vi "Telemetry2022_2.vi"() -> ()   [LabVIEW 2017]
uses:
  <vilib>/xnet/xnet.llb/XNET Frame CAN.ctl
  <vilib>/xnet/xnet.llb/XNET Frame Type CAN.ctl
  <vilib>/xnet/xnet.llb/XNET Read (Frame CAN).vi
panel:
  out "819":dbl[](array[numeric])
  out "513":dbl[](array[numeric])
  out "390":dbl[](array[numeric])
  out "389":dbl[](array[numeric])
  out "376":dbl[](array[numeric])
  out "647":dbl[](array[numeric])
  out "644":dbl[](array[numeric])
  out "645":dbl[](array[numeric])
  out "646":dbl[](array[numeric])
  out "401":dbl
  out "394":T1
  out "393":T2
  out "532":T3
  out "530":T4
  out "651":T5
  out "650":T6
  out "649":T7
  out "648":T8
  in  "ip":string="127.0.0.1"
  out "UDP timestep":u32(graph)
  out "Frames to update this timestep":u32[](array[numeric])
  in  "stresstest":bool
  out "Actual Timestep":u32(graph)
  out "105":T9
  out "1029":T10
  out "1157":T11
  out "1153":T12
  out "1030":T13
  out "873":T14
  out "820":T15
  in  "stresstest2":u8[][](array[numeric])=[[2, 132, 0, 0, 0, 0, 0, 0, 0, 0], [2, 133, 0, 0, 0, 0, 0, 0, 0, 0], [2, 134, 0, 0, 0, 0, 0, 0, 0, 0], [2, 135, 0, 0, 0, 0, 0, 0, 0, 0], [1, 116, 0, 0, 0, 0, 0, 0, 0, 0], [1, 120, 0, 0, 0, 0, 0, 0, 0, 0], [1, 133, 0, 0, 0, 0, 0, 0, 0, 0], [1, 134, 0, 0, 0, 0, 0, 0, 0, 0], [2, 1, 0, 0, 0, 0, 0, 0, 0, 0], [2, 0, 0, 0, 0, 0, 0, 0, 0, 0], [5, 129, 0, 0, 0, 0, 0, 0, 0, 0], [3, 51, 0, 0, 0, 0, 0, 0, 0, 0], [3, 52, 0, 0, 0, 0, 0, 0, 0, 0], [3, 105, 0, 0, 0, 0, 0, 0, 0, 0], [4, 6, 0, 0, 0, 0, 0, 0, 0, 0], [4, 129, 0, 0, 0, 0, 0, 0, 0, 0], [4, 133, 0, 0, 0, 0, 0, 0, 0, 0], [4, 5, 0, 0, 0, 0, 0, 0, 0, 0], [0, 105, 0, 0, 0, 0, 0, 0, 0, 0], [2, 136, 0, 0, 0, 0, 0, 0, 0, 0], [2, 137, 0, 0, 0, 0, 0, 0, 0, 0], [2, 138, 0, 0, 0, 0, 0, 0, 0, 0], [2, 139, 0, 0, 0, 0, 0, 0, 0, 0], [2, 18, 0, 0, 0, 0, 0, 0, 0, 0], [2, 20, 0, 0, 0, 0, 0, 0, 0, 0], [1, 137, 0, 0, 0, 0, 0, 0, 0, 0], [1, 138, 0, 0, 0, 0, 0, 0, 0, 0], [1, 145, 0, 0, 0, 0, 0, 0, 0, 0]]
  in  "stresstest1":u8[][](array[numeric])=[[2, 132, 1, 0, 1, 0, 1, 0, 1, 0], [2, 133, 1, 0, 1, 0, 1, 0, 1, 0], [2, 134, 1, 0, 1, 0, 1, 0, 1, 0], [2, 135, 1, 0, 1, 0, 1, 0, 1, 0], [1, 116, 0, 0, 0, 0, 1, 0, 0, 0], [1, 120, 1, 0, 0, 0, 1, 0, 0, 0], [1, 133, 0, 15, 1, 0, 1, 0, 1, 0], [1, 134, 0, 15, 1, 0, 1, 0, 1, 0], [2, 1, 1, 0, 1, 0, 1, 0, 1, 0], [2, 0, 1, 0, 1, 0, 1, 0, 1, 0], [5, 129, 1, 0, 0, 0, 0, 0, 0, 0], [3, 51, 255, 255, 255, 255, 255, 255, 255, 255], [3, 52, 255, 255, 255, 255, 255, 255, 255, 255], [3, 105, 1, 1, 1, 1, 1, 0, 0, 0], [4, 6, 0, 1, 0, 1, 0, 1, 0, 1], [4, 129, 255, 255, 255, 255, 255, 255, 255, 255], [4, 133, 255, 255, 255, 255, 255, 255, 255, 255], [4, 5, 0, 1, 0, 1, 0, 1, 0, 1], [0, 105, 0, 0, 0, 1, 1, 1, 128, 1], [2, 136, 1, 0, 1, 0, 1, 0, 1, 0], [2, 137, 1, 0, 1, 0, 1, 0, 1, 0], [2, 138, 1, 0, 1, 0, 1, 0, 1, 0], [2, 139, 1, 0, 1, 0, 1, 0, 1, 0], [2, 18, 255, 255, 255, 255, 255, 255, 255, 255], [2, 20, 1, 0, 1, 0, 1, 0, 1, 0], [1, 137, 1, 0, 1, 0, 1, 0, 1, 0], [1, 138, 1, 0, 1, 0, 1, 0, 1, 0], [1, 145, 2, 0, 0, 0, 0, 0, 0, 0]]
  out "1409":dbl
  out "512":T16
  out "372":dbl
  out "?":T17(tab)
  in  "?":bool
  out "CAN2 Frame to signal":errorcluster
  out "XNET error (CAN3)":errorcluster
  out "XNET error (CAN2)":errorcluster
  out "NI-CAN1 error":errorcluster {"code" format="%.0x"}
  out "NI-CAN0 error":errorcluster {"code" format="%.0x"}
  out "CAN1 Frame to signal":errorcluster
  out "UDP Read error":errorcluster
  in  "Data source":u16(ring) items=["WiFi-UDP", "XNET-USB", "CAN-USB", "Log Replay"]
  in  "Port":u16=23456
  in  "Main timestep":u32=10
  out "Key Navigation error":errorcluster
  out "Is running":bool
  out "Key":T18(ring)
  in  "Reset Keyboard":bool
  out "all signal data":dbl[](array[numeric])
  out "rec array":u8[][](array[numeric])=[[2, 225, 14, 196, 12, 0, 0, 0, 0, 0], [2, 226, 35, 253, 12, 0, 0, 0, 0, 0], [2, 227, 56, 248, 12, 0, 0, 0, 0, 0], [2, 228, 77, 195, 12, 0, 0, 0, 0, 0], [2, 241, 7, 28, 0, 0, 0, 0, 0, 0], [2, 242, 14, 27, 0, 0, 0, 0, 0, 0], [2, 243, 21, 29, 0, 0, 0, 0, 0, 0], [2, 244, 28, 28, 0, 0, 0, 0, 0, 0], [0, 144, 12, 42, 12, 247, 12, 20, 12, 129], [0, 112, 11, 37, 0, 225, 1, 0, 0, 0], [0, 113, 15, 104, 8, 4, 1, 0, 0, 0], [2, 0, 2, 4, 5, 5, 2, 0, 0, 0], [0, 98, 3, 242, 1, 24, 0, 131, 0, 0], [0, 99, 46, 33, 1, 1, 1, 1, 1, 44], [0, 102, 2, 71, 1, 51, 0, 74, 0, 0], [0, 103, 33, 35, 1, 1, 1, 1, 1, 44]]
  out "frame data":T19[](array[typedef]) {"payload" format="%x"; "timestamp" format="%<%.7X\n%x>T"; "type" items=["CAN Data"=0, "CAN Remote"=1, "CAN Bus Error"=2, "CAN 2.0 Data"=8, "CAN FD Data"=16, "CAN FD+BRS Data"=24, "J1939 Data"=192, "Delay"=224, "Log Trigger"=225, "Start Trigger"=226]; "identifier" format="%x"}
  # "CAN1"
  # "CAN2"
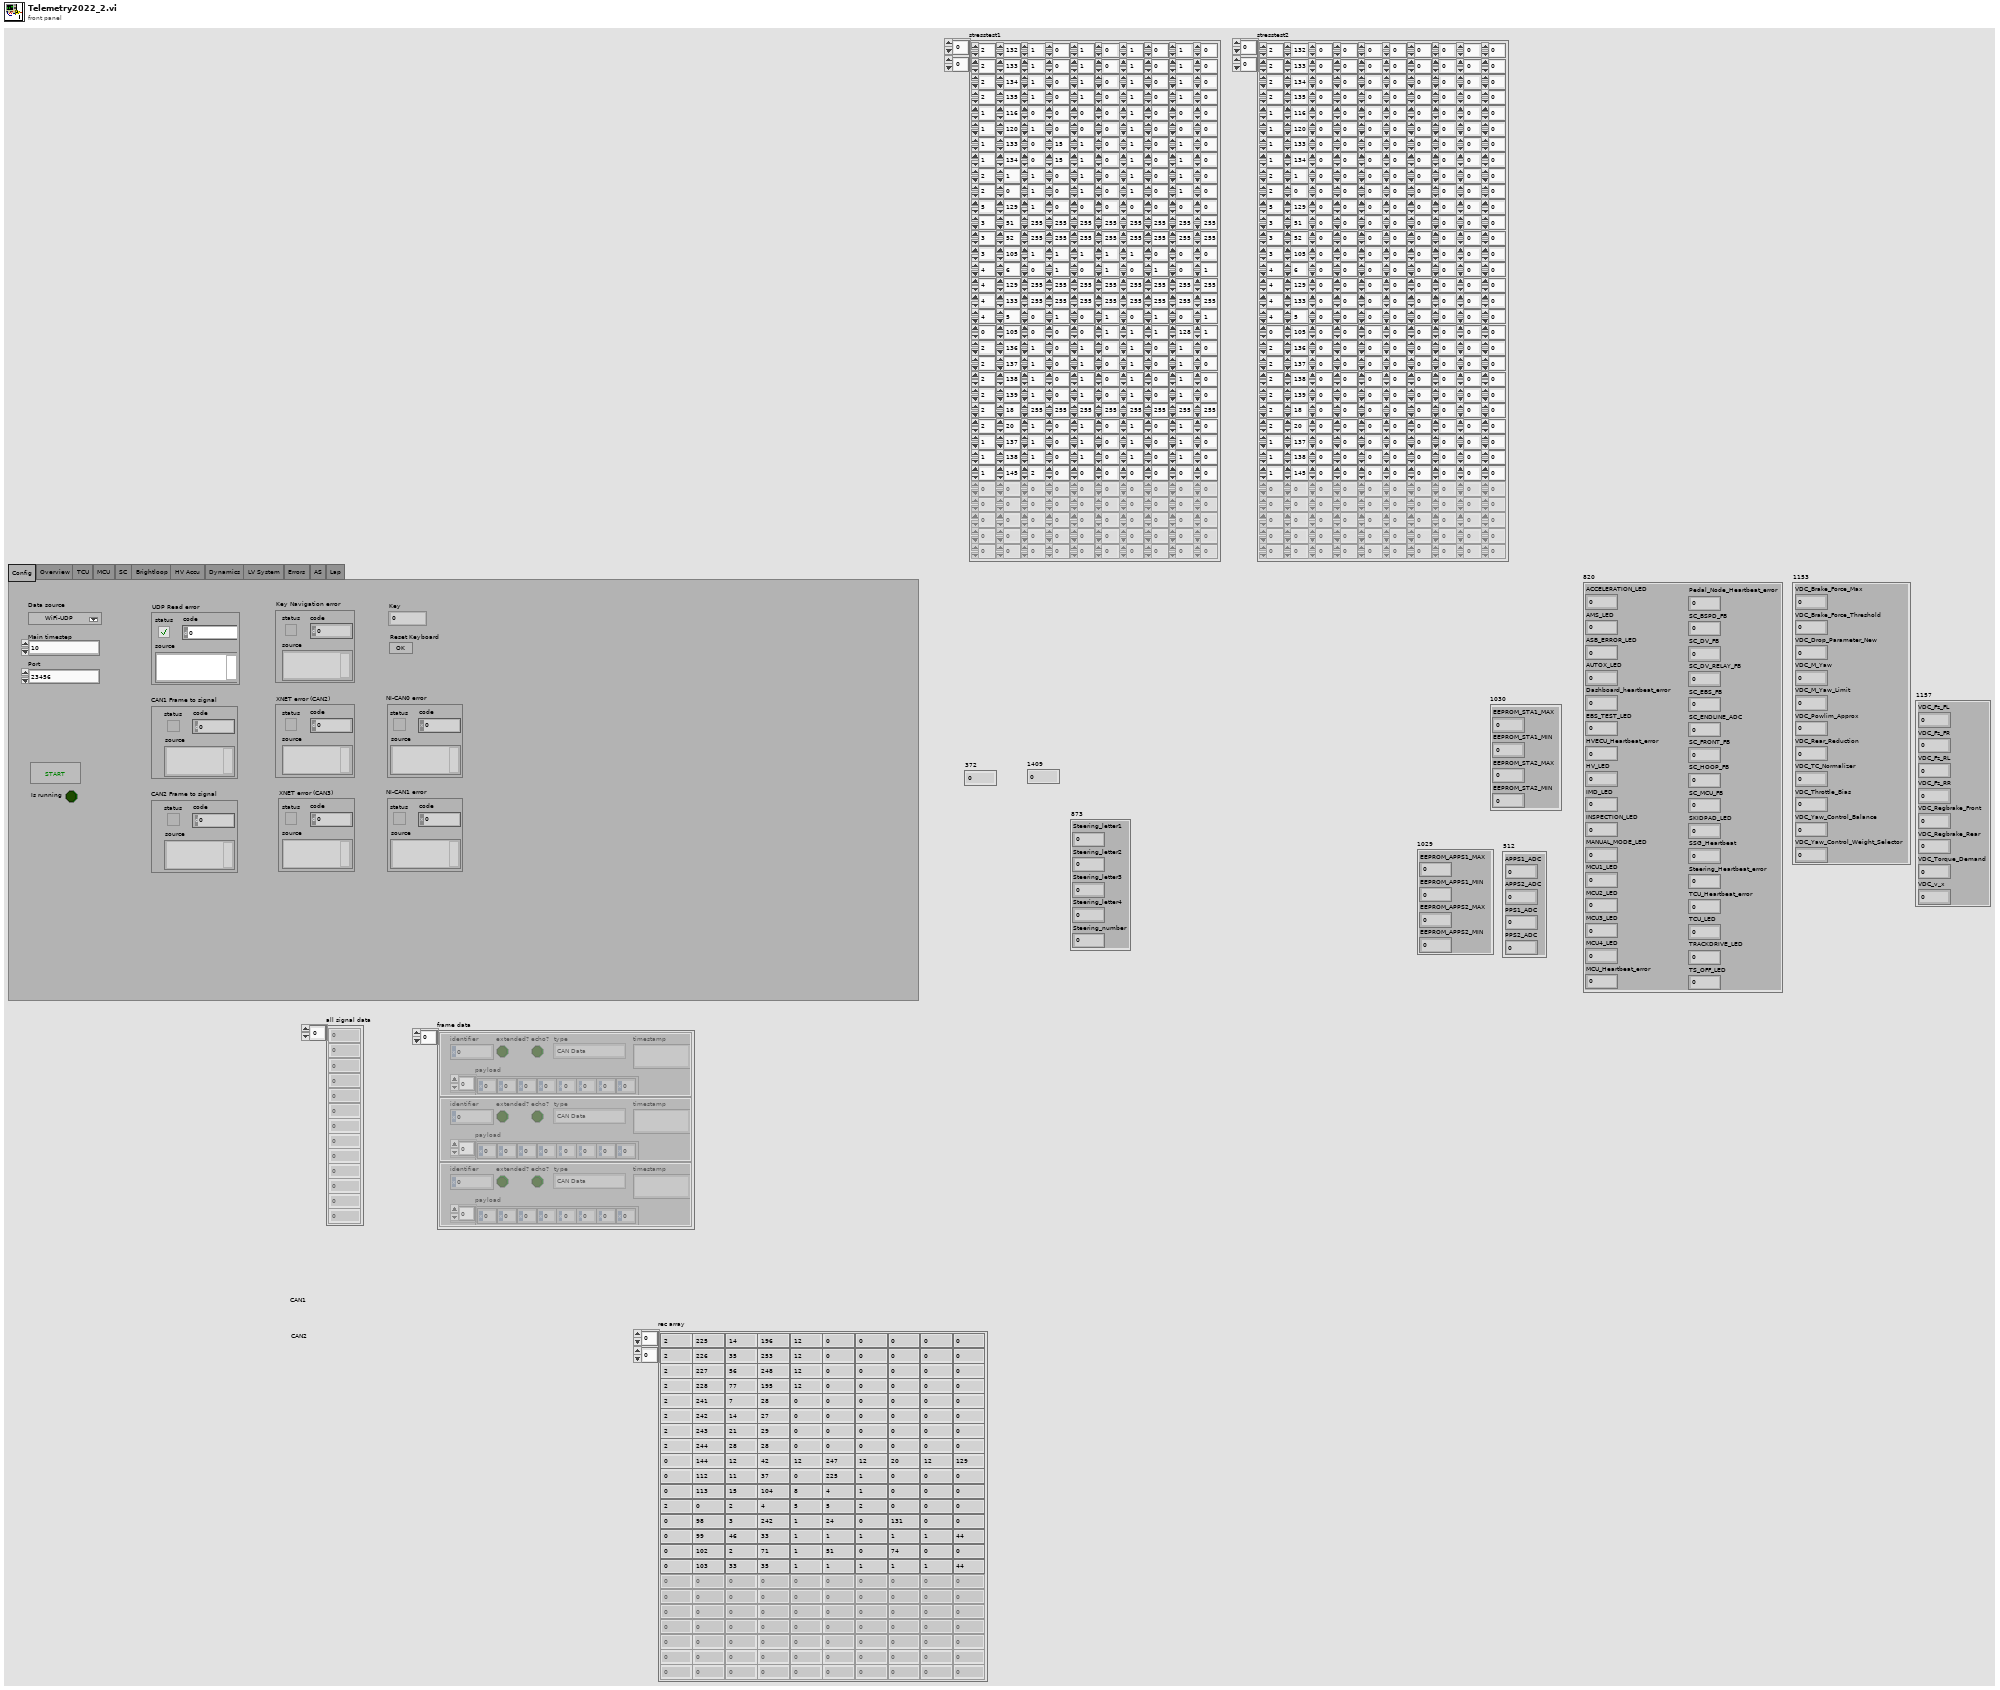
[diagram p1: front panel]
types:
  T1 = cluster{"AMK4_Control":dbl, "AMK4_Target_Velocity":dbl, "AMK4_TorqueLimitNegative":dbl, "AMK4_TorqueLimitPositive":dbl}
  T2 = cluster{"AMK3_Control":dbl, "AMK3_Target_Velocity":dbl, "AMK3_TorqueLimitNegative":dbl, "AMK3_TorqueLimitPositive":dbl}
  T3 = cluster{"HV_Current":dbl, "HV_Voltage_After_AIRs":dbl, "HV_Voltage_Before_AIRs":dbl, "State_of_Charge":dbl}
  T4 = cluster{"AIR_minus_state":dbl, "AIR_plus_State":dbl, "AMS_Relay_State":dbl, "AMS_Status":dbl, "Driver_Protection_State":dbl, "Error_STAMP_TSAL":dbl, "Error_value":dbl, "HV_Acc_Menu":dbl, "HV_Cell_OT":dbl, "HV_Cell_OV":dbl, "HV_Cell_UV":dbl, "HV_DetStatus":dbl, "HV_ECU_Heartbeat":dbl, "HV_ECU_SC_Endline_State":dbl, "IMD_Relay_State":dbl, "IMD_Status":dbl, "MCU_STAMP":dbl, "PC_Error":dbl, "PC_State":dbl, "Place_of_error":dbl, "TSAL_GREEN":dbl, "TSAL_RED":dbl, "TS_Over_Voltage":dbl, "TS_Overcurrent":dbl}
  T5 = cluster{"AMK4_error_info":dbl, "AMK4_temp_IGBT":dbl, "AMK4_temp_inverter":dbl, "AMK4_temp_motor":dbl}
  T6 = cluster{"AMK3_error_info":dbl, "AMK3_temp_IGBT":dbl, "AMK3_temp_inverter":dbl, "AMK3_temp_motor":dbl}
  T7 = cluster{"AMK4_actual_velocitiy":dbl, "AMK4_magnetizing_current":dbl, "AMK4_status":dbl, "AMK4_torque_current":dbl}
  T8 = cluster{"AMK3_actual_velocitiy":dbl, "AMK3_magnetizing_current":dbl, "AMK3_status":dbl, "AMK3_torque_current":dbl}
  T9 = cluster{"Xavier_AS_Finish":dbl, "Xavier_Target_Steering_Angle":dbl, "Xavier_Target_speed":dbl, "Xavier_heartbeat":dbl}
  T10 = cluster{"EEPROM_APPS1_MAX":dbl, "EEPROM_APPS1_MIN":dbl, "EEPROM_APPS2_MAX":dbl, "EEPROM_APPS2_MIN":dbl}
  T11 = cluster{"VDC_Fz_FL":dbl, "VDC_Fz_FR":dbl, "VDC_Fz_RL":dbl, "VDC_Fz_RR":dbl, "VDC_Regbrake_Front":dbl, "VDC_Regbrake_Rear":dbl, "VDC_Torque_Demand":dbl, "VDC_v_x":dbl}
  T12 = cluster{"VDC_Brake_Force_Max":dbl, "VDC_Brake_Force_Threshold":dbl, "VDC_Drop_Parameter_New":dbl, "VDC_M_Yaw":dbl, "VDC_M_Yaw_Limit":dbl, "VDC_Powlim_Approx":dbl, "VDC_Rear_Reduction":dbl, "VDC_TC_Normalizer":dbl, "VDC_Throttle_Bias":dbl, "VDC_Yaw_Control_Balance":dbl, "VDC_Yaw_Control_Weight_Selector":dbl}
  T13 = cluster{"EEPROM_STA1_MAX":dbl, "EEPROM_STA1_MIN":dbl, "EEPROM_STA2_MAX":dbl, "EEPROM_STA2_MIN":dbl}
  T14 = cluster{"Steering_letter1":dbl, "Steering_letter2":dbl, "Steering_letter3":dbl, "Steering_letter4":dbl, "Steering_number":dbl}
  T15 = cluster{"ACCELERATION_LED":dbl, "AMS_LED":dbl, "ASB_ERROR_LED":dbl, "AUTOX_LED":dbl, "Dashboard_heartbeat_error":dbl, "EBS_TEST_LED":dbl, "HVECU_Heartbeat_error":dbl, "HV_LED":dbl, "IMD_LED":dbl, "INSPECTION_LED":dbl, "MANUAL_MODE_LED":dbl, "MCU1_LED":dbl, "MCU2_LED":dbl, "MCU3_LED":dbl, "MCU4_LED":dbl, "MCU_Heartbeat_error":dbl, "Pedal_Node_Heartbeat_error":dbl, "SC_BSPD_FB":dbl, "SC_DV_FB":dbl, "SC_DV_RELAY_FB":dbl, "SC_EBS_FB":dbl, "SC_ENDLINE_ADC":dbl, "SC_FRONT_FB":dbl, "SC_HOOP_FB":dbl, "SC_MCU_FB":dbl, "SKIDPAD_LED":dbl, "SSG_Heartbeat":dbl, "Steering_Heartbeat_error":dbl, "TCU_Heartbeat_error":dbl, "TCU_LED":dbl, "TRACKDRIVE_LED":dbl, "TS_OFF_LED":dbl}
  T16 = cluster{"APPS1_ADC":dbl, "APPS2_ADC":dbl, "PPS1_ADC":dbl, "PPS2_ADC":dbl}
  T17 = enum32{"Config", "Overview", "TCU", "MCU", "SC", "Brightloop", "HV Accu", "Dynamics", "LV System", "Errors", "AS", "Lap"}
  T18 = enum16{"0", "1", "2", "3", "4", "5", "6", "7", "8", "9", "A", "B", "C", "D", "E", "F", "G", "H", "I", "J", "K", "L", "M", "N", "O", "P", "Q", "R", "S", "T", "U", "V", "W", "X", "Y", "Z", "F1", "F2", "F3", "F4", "F5", "F6", "F7", "F8", "F9", "F10", "F11", "F12", "F13", "F14", "F15", "ADD", "BACK", "BACKSLASH", "CAPITAL", "COMMA", "DECIMAL", "DELETE", "DIVIDE", "DOWN", "END", "EQUALS", "ESCAPE", "GRAVE (`)", "HOME", "INSERT", "LBRACKET", "LCONTROL", "LEFT", "L ALT", "LSHIFT", "LWIN", "MINUS", "MULTIPLY", "NEXT", "NUMLOCK", "NUMPAD_0", "NUMPAD_1", "NUMPAD_2", "NUMPAD_3", "NUMPAD_4", "NUMPAD_5", "NUMPAD_6", "NUMPAD_7", "NUMPAD_8", "NUMPAD_9", "PAUSE", "PERIOD", "PRIOR (PG UP)", "RBRACKET", "RCONTROL", "RETURN", "RIGHT", "R ALT", "RSHIFT", "RWIN", "SCROLL", "SEMICOLON", "SLASH", "SPACE", "SUBTRACT", "TAB", "UP", "ENTER (num pad)", "' (quote)"}
  T19 = typedef "XNET Frame CAN.ctl" = cluster{"timestamp":timestamp, "payload":u8[], "identifier":u32, "type":T20, "extended?":bool, "echo?":bool}
  T20 = typedef "XNET Frame Type CAN.ctl" = u8
  T21 = cluster{"XNET session A":refnum<k21>, "Error out A ":errorcluster, "XNET session B":refnum<k21>, "Error out B":errorcluster}
  T22 = typedef "xobjhandle.ctl" = u32
  T23 = cluster{"ObjHandle A":T22, "Error out A":errorcluster, "ObjHandle B":T22, "Error out B":errorcluster}
  T24 = cluster{"Signal count":i32, "Conversion session":refnum<k21>, "Conversion error":errorcluster}
  T25 = cluster{"Brake_Force_sensor":dbl, "Brake_force_validity":dbl, "Brake_pressure_front":dbl, "Brake_pressure_front_validity":dbl, "Brake_pressure_rear":dbl, "Brake_pressure_rear_validity":dbl, "SC_ENDLINE":dbl}
  T26 = cluster{"ASF_BFS_Vectornav_12V":dbl, "ASMS":dbl, "ASSI_state":dbl, "AS_GO_Signal":dbl, "AS_Mission_selected":dbl, "Brake_Light":dbl, "Buzzer":dbl, "CAN_Nodes_24V":dbl, "Calibration_Enabled":dbl, "Calibration_State":dbl, "Can_Nodes_Configured":dbl, "Datalogger_2D_12V":dbl, "Driving_State_Active":dbl, "EBS_FB":dbl, "EBS_IS_ACTIVE":dbl, "External_TS_Button":dbl, "Initial_Checkup_state":dbl, "MCU_EF_State":dbl, "MCU_FRONT_SUPPLY":dbl, "MCU_REAR_SUPPLY":dbl, "MCU_RF_State":dbl, "OFF_Car_State":dbl, "ON_Car_State":dbl, "PPS1":dbl, "PPS2":dbl, "Pump":dbl, "RTDS":dbl, "SB_ENGAGE":dbl, "SB_FB":dbl, "SC_Close":dbl, "SC_START":dbl, "SET_FINISH_STATE":dbl, "START_Car_State":dbl, "TCU_Power":dbl, "WATCHDOG":dbl, "Xavier_12V":dbl, "nEBS_ENGAGE":dbl, "nEBS_IS_TRIGGERED":dbl, "nEBS_SET_ACTIVE":dbl, "nSet_Driving_State":dbl}
  T27 = cluster{"Button1":dbl, "Button2":dbl, "Button3":dbl, "Button4":dbl, "Rotary1":dbl, "Rotary2":dbl, "Rotary3":dbl, "Rotary4":dbl, "Rotary5":dbl, "Steering_heartbeat":dbl}
  T28 = cluster{"APPS1_position":dbl, "APPS1_validity":dbl, "APPS2_posiition":dbl, "APPS2_validity":dbl, "APPS_plausiblity":dbl, "STA1_position":dbl, "STA1_validity":dbl, "STA2_position":dbl, "STA2_validity":dbl, "STA_plausiblity":dbl}
  T29 = cluster{"Button_OFF":dbl, "Button_ON":dbl, "Button_START":dbl, "Dash_BLANK":dbl, "Dash_MODE":dbl, "Dash_XLAT":dbl, "Dashboard_ID":dbl, "Dashboarrd_heartbeat":dbl}
  T30 = cluster{"HV_Current":dbl, "HV_Voltage_After_AIRs":dbl, "HV_Voltage_Before_AIRs":dbl}
  T31 = cluster{"AMK1_actual_velocitiy":dbl, "AMK1_magnetizing_current":dbl, "AMK1_status":dbl, "AMK1_torque_current":dbl}
  T32 = cluster{"AMK2_actual_velocitiy":dbl, "AMK2_magnetizing_current":dbl, "AMK2_status":dbl, "AMK2_torque_current":dbl}
  T33 = cluster{"AMK1_error_info":dbl, "AMK1_temp_IGBT":dbl, "AMK1_temp_inverter":dbl, "AMK1_temp_motor":dbl}
  T34 = cluster{"AMK2_error_info":dbl, "AMK2_temp_IGBT":dbl, "AMK2_temp_inverter":dbl, "AMK2_temp_motor":dbl}
  T35 = cluster{"ASF_X_Acceleration":dbl, "ASF_Yaw_rate":dbl}
  T36 = cluster{"AMK1_DC_ON":dbl, "AMK1_Enable":dbl, "AMK1_Error_Reset":dbl, "AMK1_Inverter_On":dbl, "AMK1_Target_Velocity":dbl, "AMK1_Torque_Limit_Negative":dbl, "AMK1_Torque_Limit_Positive":dbl}
  T37 = cluster{"AMK2_DC_ON":dbl, "AMK2_Enable":dbl, "AMK2_Error_Reset":dbl, "AMK2_Inverter_On":dbl, "AMK2_Target_Velocity":dbl, "AMK2_Torque_Limit_Negative":dbl, "AMK2_Torque_Limit_Positive":dbl}
  T38 = cluster{"Brake_pressure_front_ADC":dbl, "Brake_pressure_rear_ADC":dbl, "STA1_ADC":dbl, "STA2_ADC":dbl}
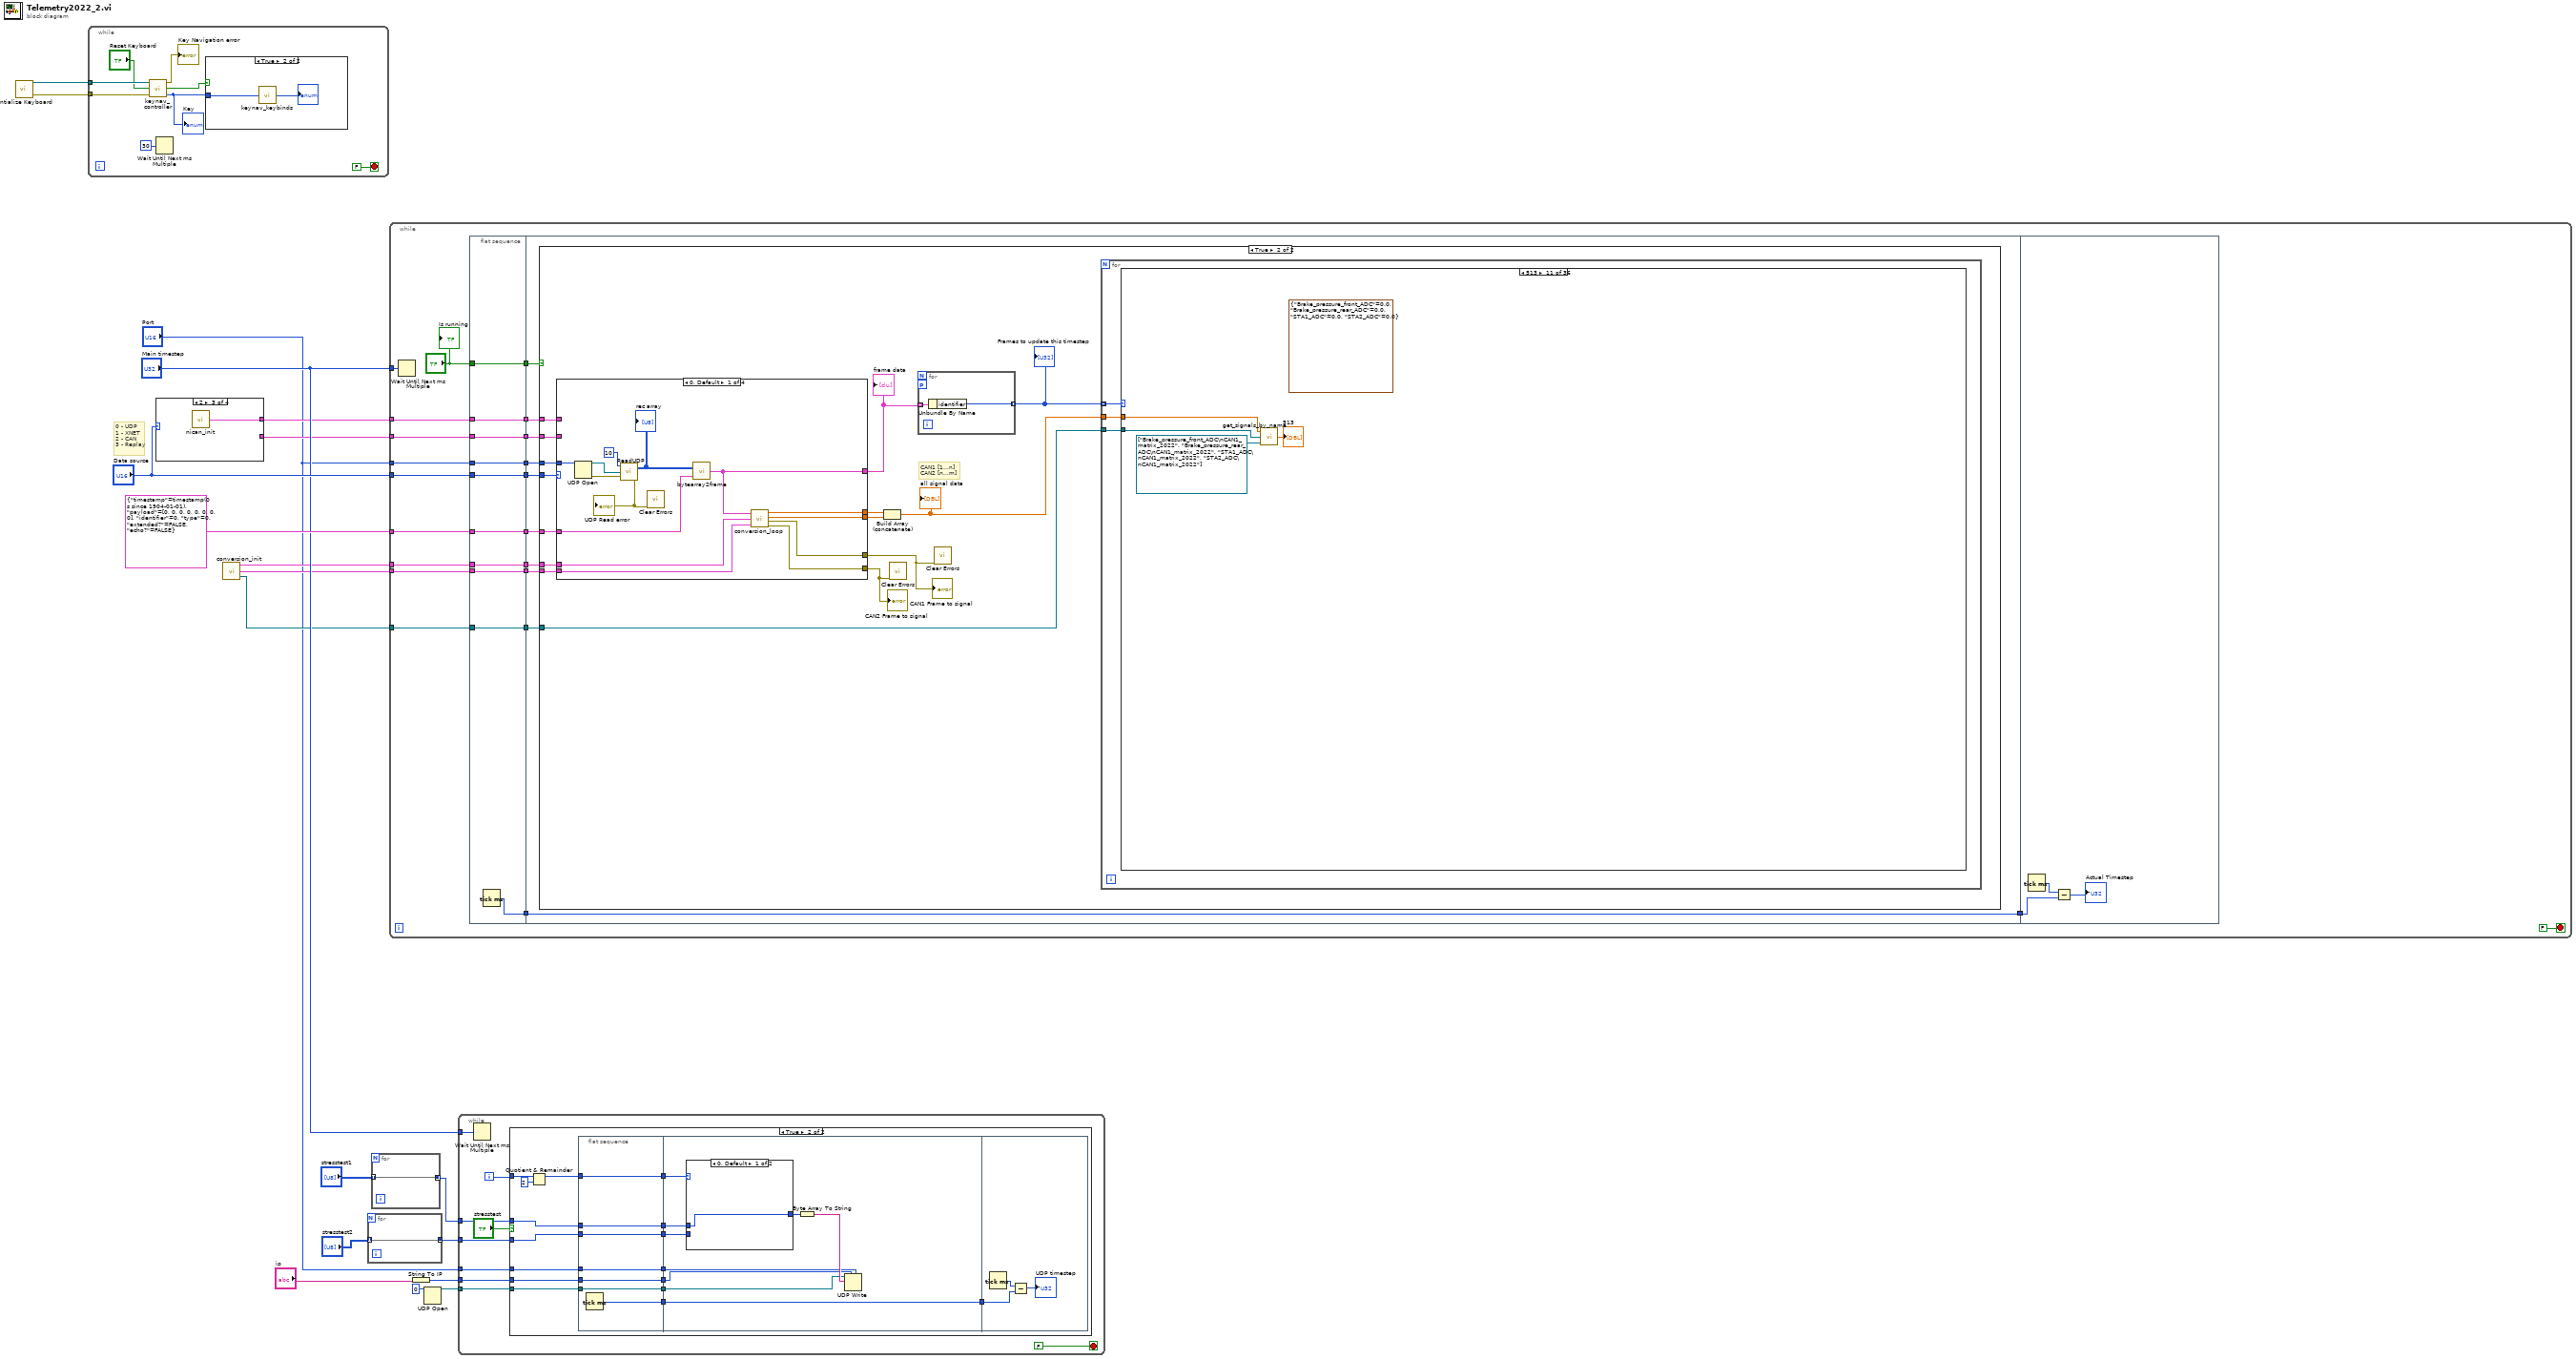
[diagram p0: block diagram]
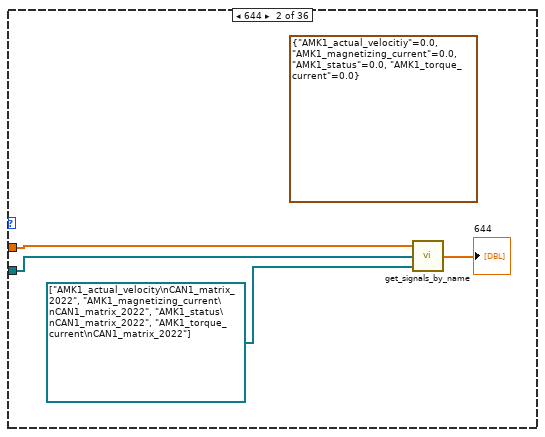
[diagram p7: hidden frame]
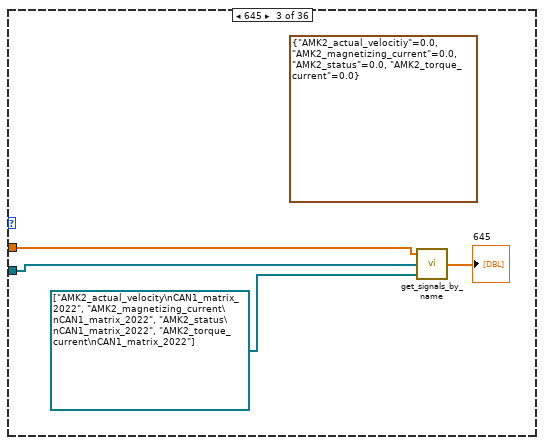
[diagram p8: hidden frame]
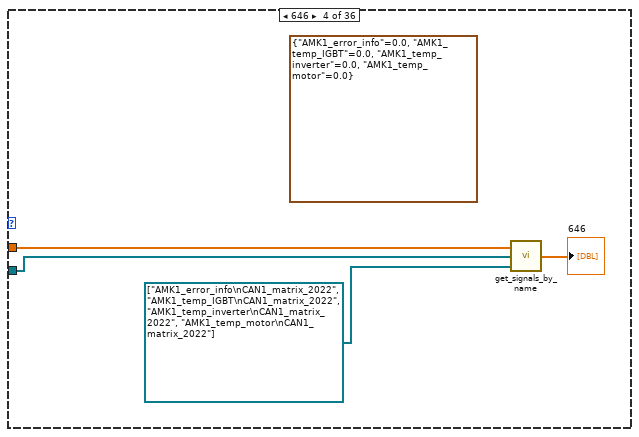
[diagram p9: hidden frame]
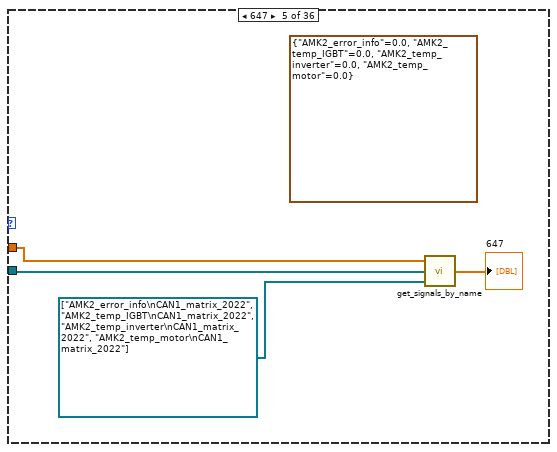
[diagram p10: hidden frame]
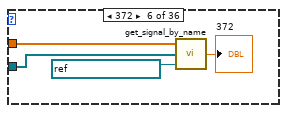
[diagram p11: hidden frame]
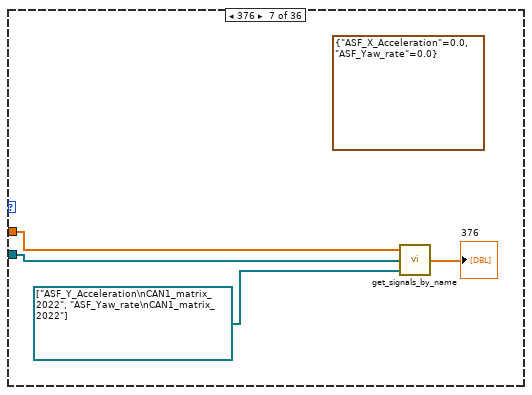
[diagram p12: hidden frame]
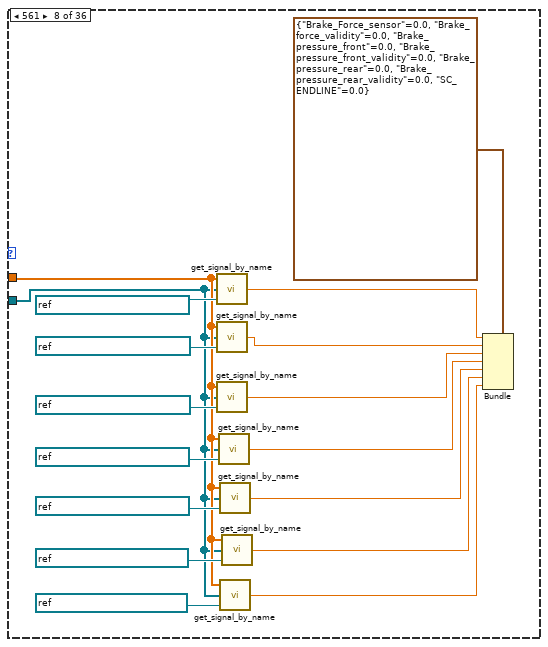
[diagram p13: hidden frame]
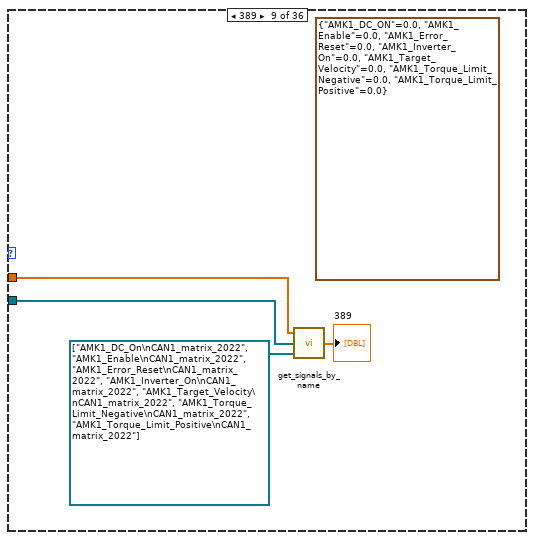
[diagram p14: hidden frame]
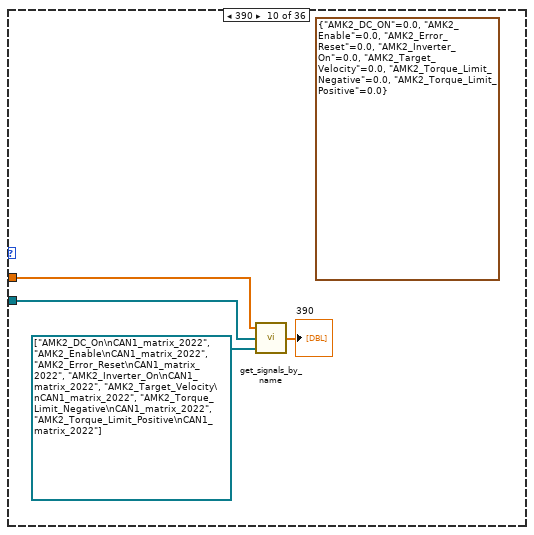
[diagram p15: hidden frame]
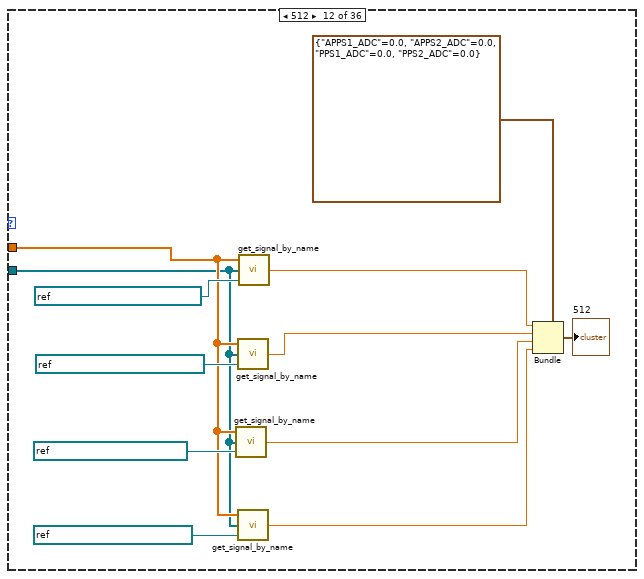
[diagram p16: hidden frame]
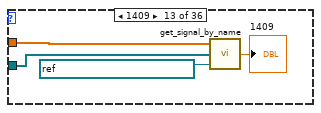
[diagram p17: hidden frame]
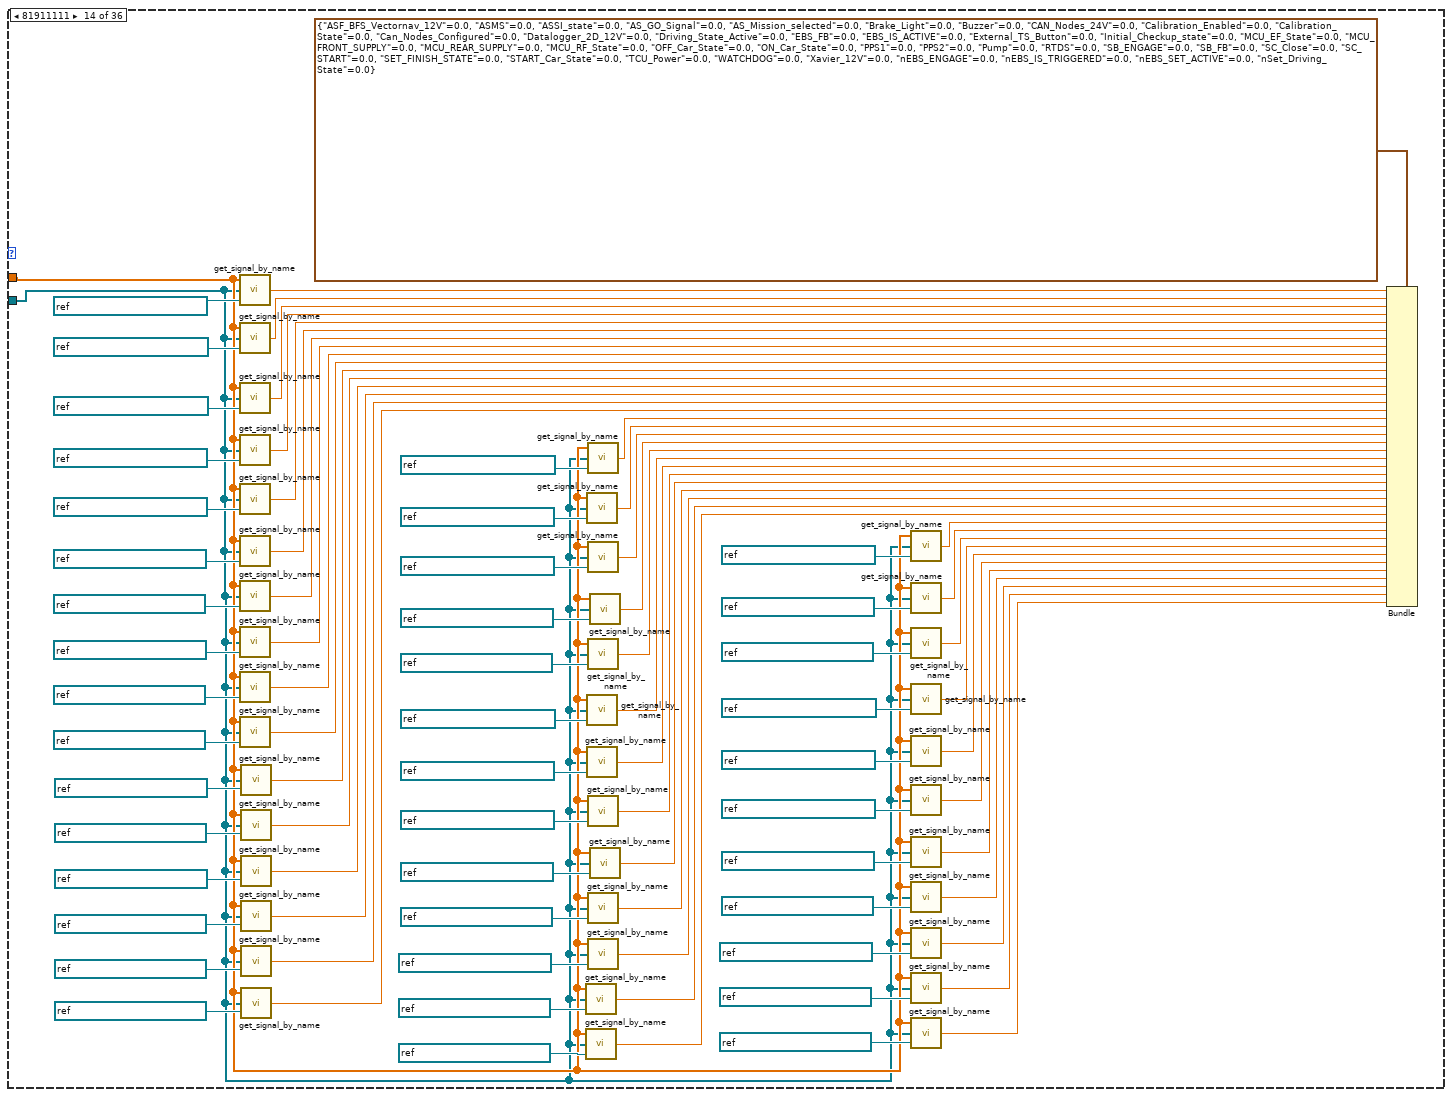
[diagram p18: hidden frame]
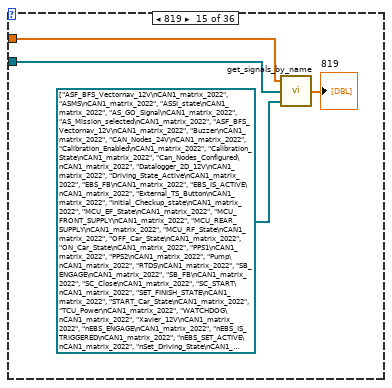
[diagram p19: hidden frame]
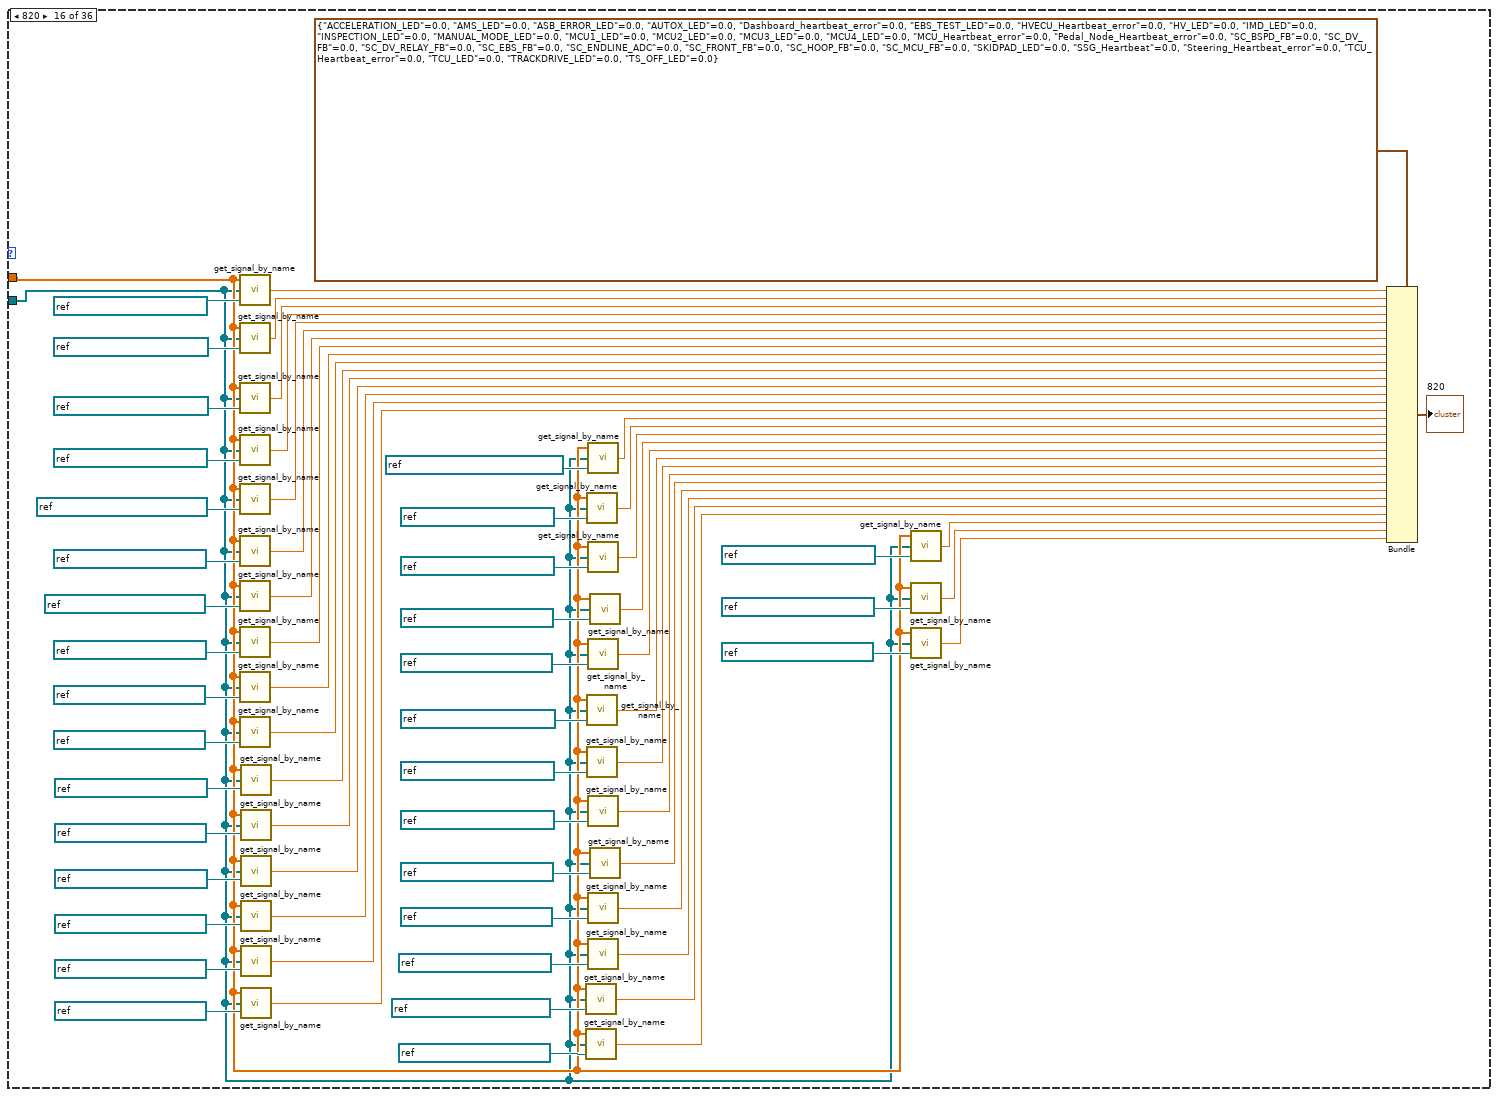
[diagram p20: hidden frame]
diagram:
  # "0 - UDP\n1 - XNET\n2 - CAN\n3 - Replay"
  n1 = call <vilib>:"Intialize Keyboard.vi"() -> ("error out"=w6:errorcluster, "device ID"=w7:refnum<k1>)  [unwired: 10 in]
  n2 = while {
    tunnel: w7 -> [w26]
    tunnel: w6 -> [w25]
    stop <- FALSE stop-if-true
    n3 = call "keynav_controller.vi"("Error in"=w25, "Reset Keyboard"="Reset Keyboard", "Keyboard id"=w26) -> ("Key"=w22:T18, "Enable"=w23:bool, "Keynav error"=→"Key Navigation error":errorcluster)
    "Key" <- w22
    n4 = Wait Until Next ms Multiple(millisecond multiple=u32 30) -> ()  [unwired: 1 out]
    n5 = case shown="True" w23 {
      tunnel: w22 -> [_ w29]
      frame False {
      }
      frame True {
        n6 = call "keynav_keybinds.vi"("Key"=w29) -> ("Tab id"=→"?":i32)
      }
    }
  }
  n7 = case shown="2" "Data source" {
    tunnel: [_ _ w31 _] -> w12
    tunnel: [_ w30 _ _] -> w11
    frame 0, Default {
    }
    frame 1 {
      n8 = call "xnet_init.vi"() -> ("XNET Init"=w30:T21)  [unwired: 1 in]
    }
    frame 2 {
      n9 = call "nican_init.vi"() -> ("CAN Init"=w31:T23)  [unwired: 2 in]
    }
    frame 3 {
    }
  }
  n10 = call "conversion_init.vi"() -> ("Signal list"=w10:refnum<k21>[], "CAN2 conversion session"=w9:T24, "CAN1 conversion session"=w8:T24)
  n11 = for {
    tunnel: "stresstest2" -> [w32] mode=indexing
    tunnel: [w32] -> w14 mode=concatenating
  }
  n12 = for {
    tunnel: "stresstest1" -> [w33] mode=indexing
    tunnel: [w33] -> w16 mode=concatenating
  }
  n13 = while {
    tunnel: "Port" -> [w55]
    tunnel: "Data source" -> [w54]
    tunnel: T19 {"timestamp"=timestamp(0 s since 1904-01-01), "payload"=[0, 0, 0, 0, 0, 0, 0, 0], "identifier"=0, "type"=0, "extended?"=FALSE, "echo?"=FALSE} ("CAN frame") -> [w53]
    tunnel: "Main timestep" -> [w52]
    tunnel: w10 -> [w49]
    tunnel: w12 -> [w41]
    tunnel: w11 -> [w38]
    tunnel: w9 -> [w36]
    tunnel: w8 -> [w34]
    stop <- FALSE stop-if-true
    n14 = Wait Until Next ms Multiple(millisecond multiple=w52) -> ()  [unwired: 1 out]
    n15 = flat-sequence {
      tunnel: w49 -> [w61]
      tunnel: "?" -> [w62]
      tunnel: w53 -> [w63]
      tunnel: w54 -> [w64]
      tunnel: w55 -> [w65]
      tunnel: [w65] -> w48
      tunnel: [w64] -> w47
      tunnel: [w63] -> w46
      tunnel: [w62] -> w45
      tunnel: [w61] -> w44
      tunnel: [w60] -> w43
      tunnel: w41 -> [w59]
      tunnel: [w59] -> w40
      tunnel: [w58] -> w39
      tunnel: w38 -> [w58]
      tunnel: [w57] -> w37
      tunnel: w36 -> [w57]
      tunnel: [w56] -> w35
      tunnel: w34 -> [w56]
      tunnel: w48 -> [w75]
      tunnel: w47 -> [w74]
      tunnel: w46 -> [w73]
      tunnel: w45 -> [w72]
      tunnel: w44 -> [w71]
      tunnel: w43 -> [w70]
      tunnel: [w70] -> w42
      tunnel: w40 -> [w69]
      tunnel: w39 -> [w68]
      tunnel: w37 -> [w66]
      tunnel: w35 -> [w67]
      tunnel: w42 -> [w690]
      frame #0 {
        n16 = Tick Count (ms)() -> (millisecond timer value=w60:u32)
      }
      frame #1 {
        n17 = case shown="True" w72 {
          tunnel: w75 -> [_ w90]
          tunnel: w74 -> [_ w89]
          tunnel: w73 -> [_ w88]
          tunnel: w71 -> [_ w81]
          tunnel: w69 -> [_ w79]
          tunnel: w68 -> [_ w78]
          tunnel: w67 -> [_ w77]
          tunnel: w66 -> [_ w76]
          frame False {
          }
          frame True {
            # "CAN1 [1...n]\nCAN2 [n...m]"
            n18 = case shown="0, Default" w89 {
              tunnel: w90 -> [w650 _ _ _]
              tunnel: w88 -> [w641 _ w676 w686]
              tunnel: [w643 w659 w675 w687] -> w83
              tunnel: [w647 w656 w674 w684] -> w86
              tunnel: [w646 w655 w673 w684] -> w87
              tunnel: [w645 w653 w671 w685] -> w85
              tunnel: [w644 w654 w672 w685] -> w84
              tunnel: w79 -> [_ _ w681 _]
              tunnel: w78 -> [_ w664 _ _]
              tunnel: w77 -> [w640 w657 w670 _]
              tunnel: w76 -> [w639 w658 w669 _]
              frame 0, Default {
                n19 = UDP Open(11:w650) -> (port=w648:refnum<k16>, 0:w649:errorcluster)  [unwired: 4 in, 1 out]
                n20 = call "ReadUDP.vi"("error in (no error)"=w649, "connection ID"=w648, "Message length"=u16 10) -> ("error out"=w652:errorcluster, "Array"=w642:u8[][])
                "rec array" <- w642
                "UDP Read error" <- w652
                n21 = call <vilib>:"Clear Errors.vi"("error in (no error)"=w652) -> ()  [unwired: 5 in, 2 out]
                n22 = call "bytearray2frame.vi"("CAN template"=w641, "2D Array"=w642) -> ("CAN frame array"=w643:T19[])
                n23 = call "conversion_loop.vi"("CAN frame array"=w643, "CAN1 conversion session"=w640, "CAN2 conversion session"=w639) -> ("CAN1 signal data"=w647:dbl[], "CAN2 signal data"=w646:dbl[], "CAN1 error out"=w644:errorcluster, "CAN2 error out"=w645:errorcluster)  [unwired: 2 in]
              }
              frame 1 {
                n24 = Unbundle(w664) -> ("XNET session A"=w663:refnum<k21>, "Error out A"=w662:errorcluster, "XNET session B"=w661:refnum<k21>, "Error out B"=w660:errorcluster)
                n25 = call-poly <vilib>:"XNET Read.vi"("session in"=w661, "error in (no error)"=w660) -> ("data"=w666:T19[], "error out"=w667:errorcluster)  [unwired: 10 in, 2 out]
                "XNET error (CAN3)" <- w667
                n26 = call-poly <vilib>:"XNET Read.vi"("session in"=w663, "error in (no error)"=w662) -> ("data"=w665:T19[], "error out"=w668:errorcluster)  [unwired: 10 in, 2 out]
                "XNET error (CAN2)" <- w668
                n27 = call <vilib>:"Clear Errors.vi"("error in (no error)"=w667) -> ()  [unwired: 5 in, 2 out]
                n28 = Build Array (concatenate)(w665, w666) -> (w659:T19[])
                n29 = call <vilib>:"Clear Errors.vi"("error in (no error)"=w668) -> ()  [unwired: 5 in, 2 out]
                n30 = call "conversion_loop.vi"("CAN frame array"=w659, "CAN1 conversion session"=w657, "CAN2 conversion session"=w658) -> ("CAN1 signal data"=w656:dbl[], "CAN2 signal data"=w655:dbl[], "CAN1 error out"=w654:errorcluster, "CAN2 error out"=w653:errorcluster)  [unwired: 2 in]
              }
              frame 2 {
                n31 = Unbundle(w681) -> ("ObjHandle A"=w680:T22, "Error out A"=w679:errorcluster, "ObjHandle B"=w678:T22, "Error out B"=w677:errorcluster)
                n32 = call "nican_loop.vi"("ObjHandle A"=w680, "Error in A"=w679, "ObjHandle B"=w678, "CAN template"=w676, "Error in B"=w677) -> ("Error out A"=w683:errorcluster, "Frames read"=w675:T19[], "Error out B"=w682:errorcluster)  [unwired: 1 in]
                "NI-CAN0 error" <- w683
                "NI-CAN1 error" <- w682
                n33 = call <vilib>:"Clear Errors.vi"("error in (no error)"=w682) -> ()  [unwired: 5 in, 2 out]
                n34 = call <vilib>:"Clear Errors.vi"("error in (no error)"=w683) -> ()  [unwired: 5 in, 2 out]
                n35 = call "conversion_loop.vi"("CAN frame array"=w675, "CAN1 conversion session"=w670, "CAN2 conversion session"=w669) -> ("CAN1 signal data"=w674:dbl[], "CAN2 signal data"=w673:dbl[], "CAN1 error out"=w672:errorcluster, "CAN2 error out"=w671:errorcluster)  [unwired: 2 in]
              }
              frame 3 {
                w685 = errorcluster {"status"=FALSE, "code"=0, "source"=""} ("error out")
                w684 = dbl[] [] ("signal data")
                n36 = Build Array(w686) -> (w687:T19[])
              }
            }
            "CAN1 Frame to signal" <- w84
            "frame data" <- w83
            "CAN2 Frame to signal" <- w85
            n37 = Build Array (concatenate)(w86, w87) -> (w82:dbl[])
            "all signal data" <- w82
            n38 = call <vilib>:"Clear Errors.vi"("error in (no error)"=w85) -> ()  [unwired: 5 in, 2 out]
            n39 = for {
              tunnel: w83 -> [w638] mode=indexing
              tunnel: [w637] -> w80 mode=indexing
              workers-P: _ -> [_]
              n40 = Unbundle By Name(w638) -> ("identifier"=w637:u32)
            }
            "Frames to update this timestep" <- w80
            n41 = call <vilib>:"Clear Errors.vi"("error in (no error)"=w84) -> ()  [unwired: 5 in, 2 out]
            n42 = for {
              tunnel: w80 -> [w93] mode=indexing
              tunnel: w82 -> [w92]
              tunnel: w81 -> [w91]
              n43 = case shown="513" w93 {
                tunnel: w92 -> [_ w95 w98 w105 w106 w113 w114 w126 w136 w139 w143 w149 w161 w175 w247 w255 w321 w334 w348 w370 w395 w415 w426 w449 w466 w478 w490 w502 w517 w540 w581 w592 w601 w611 w623 w636]
                tunnel: w91 -> [_ w96 w99 w103 w107 w112 w115 w125 w137 w140 w144 w148 w160 w174 w248 w254 w320 w333 w347 w369 w394 w414 w425 w450 w465 w477 w489 w501 w516 w541 w580 w591 w600 w610 w622 w635]
                frame 0, Default {
                }
                frame 644 {
                  (unwired) T31 {"AMK1_actual_velocitiy"=0.0, "AMK1_magnetizing_current"=0.0, "AMK1_status"=0.0, "AMK1_torque_current"=0.0}
                  n44 = call "get_signals_by_name.vi"("Signals to read"=refnum<k21>[] ["AMK1_actual_velocity\nCAN1_matrix_2022", "AMK1_magnetizing_current\nCAN1_matrix_2022", "AMK1_status\nCAN1_matrix_2022", "AMK1_torque_current\nCAN1_matrix_2022"] ("Signal list"), "Signal list"=w96, "Signal data"=w95) -> ("Signals"=→"644":dbl[])
                }
                frame 645 {
                  (unwired) T32 {"AMK2_actual_velocitiy"=0.0, "AMK2_magnetizing_current"=0.0, "AMK2_status"=0.0, "AMK2_torque_current"=0.0}
                  n45 = call "get_signals_by_name.vi"("Signals to read"=refnum<k21>[] ["AMK2_actual_velocity\nCAN1_matrix_2022", "AMK2_magnetizing_current\nCAN1_matrix_2022", "AMK2_status\nCAN1_matrix_2022", "AMK2_torque_current\nCAN1_matrix_2022"] ("Signal list"), "Signal list"=w99, "Signal data"=w98) -> ("Signals"=→"645":dbl[])
                }
                frame 646 {
                  (unwired) T33 {"AMK1_error_info"=0.0, "AMK1_temp_IGBT"=0.0, "AMK1_temp_inverter"=0.0, "AMK1_temp_motor"=0.0}
                  n46 = call "get_signals_by_name.vi"("Signals to read"=refnum<k21>[] ["AMK1_error_info\nCAN1_matrix_2022", "AMK1_temp_IGBT\nCAN1_matrix_2022", "AMK1_temp_inverter\nCAN1_matrix_2022", "AMK1_temp_motor\nCAN1_matrix_2022"] ("Signal list"), "Signal list"=w103, "Signal data"=w105) -> ("Signals"=→"646":dbl[])
                }
                frame 647 {
                  (unwired) T34 {"AMK2_error_info"=0.0, "AMK2_temp_IGBT"=0.0, "AMK2_temp_inverter"=0.0, "AMK2_temp_motor"=0.0}
                  n47 = call "get_signals_by_name.vi"("Signals to read"=refnum<k21>[] ["AMK2_error_info\nCAN1_matrix_2022", "AMK2_temp_IGBT\nCAN1_matrix_2022", "AMK2_temp_inverter\nCAN1_matrix_2022", "AMK2_temp_motor\nCAN1_matrix_2022"] ("Signal list"), "Signal list"=w107, "Signal data"=w106) -> ("Signals"=→"647":dbl[])
                }
                frame 372 {
                  n48 = call "get_signal_by_name.vi"("Signal name"=refnum<k21> "ASF_X_Acceleration\nCAN1_matrix_2022", "Signal list"=w112, "Signal data"=w113) -> ("Signal"=→"372":dbl)
                }
                frame 376 {
                  (unwired) T35 {"ASF_X_Acceleration"=0.0, "ASF_Yaw_rate"=0.0}
                  n49 = call "get_signals_by_name.vi"("Signals to read"=refnum<k21>[] ["ASF_Y_Acceleration\nCAN1_matrix_2022", "ASF_Yaw_rate\nCAN1_matrix_2022"] ("Signal list"), "Signal list"=w115, "Signal data"=w114) -> ("Signals"=→"376":dbl[])
                }
                frame 561 {
                  n50 = call "get_signal_by_name.vi"("Signal name"=refnum<k21> "Brake_Force_sensor\nCAN1_matrix_2022", "Signal list"=w125, "Signal data"=w126) -> ("Signal"=w124:dbl)
                  n51 = call "get_signal_by_name.vi"("Signal name"=refnum<k21> "Brake_force_validity\nCAN1_matrix_2022", "Signal list"=w125, "Signal data"=w126) -> ("Signal"=w123:dbl)
                  n52 = call "get_signal_by_name.vi"("Signal name"=refnum<k21> "Brake_pressure_front\nCAN1_matrix_2022", "Signal list"=w125, "Signal data"=w126) -> ("Signal"=w118:dbl)
                  n53 = call "get_signal_by_name.vi"("Signal name"=refnum<k21> "Brake_pressure_front_validity\nCAN1_matrix_2022", "Signal list"=w125, "Signal data"=w126) -> ("Signal"=w119:dbl)
                  n54 = call "get_signal_by_name.vi"("Signal name"=refnum<k21> "Brake_pressure_rear\nCAN1_matrix_2022", "Signal list"=w125, "Signal data"=w126) -> ("Signal"=w120:dbl)
                  n55 = call "get_signal_by_name.vi"("Signal name"=refnum<k21> "SC_ENDLINE\nCAN1_matrix_2022", "Signal list"=w125, "Signal data"=w126) -> ("Signal"=w122:dbl)
                  n56 = call "get_signal_by_name.vi"("Signal name"=refnum<k21> "Brake_pressure_rear_validity\nCAN1_matrix_2022", "Signal list"=w125, "Signal data"=w126) -> ("Signal"=w121:dbl)
                  n57 = Bundle(cluster=T25 {"Brake_Force_sensor"=0.0, "Brake_force_validity"=0.0, "Brake_pressure_front"=0.0, "Brake_pressure_front_validity"=0.0, "Brake_pressure_rear"=0.0, "Brake_pressure_rear_validity"=0.0, "SC_ENDLINE"=0.0}, "Brake_Force_sensor"=w124, "Brake_force_validity"=w123, "Brake_pressure_front"=w118, "Brake_pressure_front_validity"=w119, "Brake_pressure_rear"=w120, "Brake_pressure_rear_validity"=w121, "SC_ENDLINE"=w122) -> ()  [unwired: 1 out]
                }
                frame 389 {
                  (unwired) T36 {"AMK1_DC_ON"=0.0, "AMK1_Enable"=0.0, "AMK1_Error_Reset"=0.0, "AMK1_Inverter_On"=0.0, "AMK1_Target_Velocity"=0.0, "AMK1_Torque_Limit_Negative"=0.0, "AMK1_Torque_Limit_Positive"=0.0}
                  n58 = call "get_signals_by_name.vi"("Signals to read"=refnum<k21>[] ["AMK1_DC_On\nCAN1_matrix_2022", "AMK1_Enable\nCAN1_matrix_2022", "AMK1_Error_Reset\nCAN1_matrix_2022", "AMK1_Inverter_On\nCAN1_matrix_2022", "AMK1_Target_Velocity\nCAN1_matrix_2022", "AMK1_Torque_Limit_Negative\nCAN1_matrix_2022", "AMK1_Torque_Limit_Positive\nCAN1_matrix_2022"], "Signal list"=w137, "Signal data"=w136) -> ("Signals"=→"389":dbl[])
                }
                frame 390 {
                  (unwired) T37 {"AMK2_DC_ON"=0.0, "AMK2_Enable"=0.0, "AMK2_Error_Reset"=0.0, "AMK2_Inverter_On"=0.0, "AMK2_Target_Velocity"=0.0, "AMK2_Torque_Limit_Negative"=0.0, "AMK2_Torque_Limit_Positive"=0.0}
                  n59 = call "get_signals_by_name.vi"("Signals to read"=refnum<k21>[] ["AMK2_DC_On\nCAN1_matrix_2022", "AMK2_Enable\nCAN1_matrix_2022", "AMK2_Error_Reset\nCAN1_matrix_2022", "AMK2_Inverter_On\nCAN1_matrix_2022", "AMK2_Target_Velocity\nCAN1_matrix_2022", "AMK2_Torque_Limit_Negative\nCAN1_matrix_2022", "AMK2_Torque_Limit_Positive\nCAN1_matrix_2022"], "Signal list"=w140, "Signal data"=w139) -> ("Signals"=→"390":dbl[])
                }
                frame 513 {
                  (unwired) T38 {"Brake_pressure_front_ADC"=0.0, "Brake_pressure_rear_ADC"=0.0, "STA1_ADC"=0.0, "STA2_ADC"=0.0}
                  n60 = call "get_signals_by_name.vi"("Signals to read"=refnum<k21>[] ["Brake_pressure_front_ADC\nCAN1_matrix_2022", "Brake_pressure_rear_ADC\nCAN1_matrix_2022", "STA1_ADC\nCAN1_matrix_2022", "STA2_ADC\nCAN1_matrix_2022"], "Signal list"=w144, "Signal data"=w143) -> ("Signals"=→"513":dbl[])
                }
                frame 512 {
                  n61 = call "get_signal_by_name.vi"("Signal name"=refnum<k21> "PPS1_ADC\nCAN1_matrix_2022", "Signal list"=w148, "Signal data"=w149) -> ("Signal"=w151:dbl)
                  n62 = call "get_signal_by_name.vi"("Signal name"=refnum<k21> "APPS2_ADC\nCAN1_matrix_2022", "Signal list"=w148, "Signal data"=w149) -> ("Signal"=w150:dbl)
                  n63 = call "get_signal_by_name.vi"("Signal name"=refnum<k21> "PPS2_ADC\nCAN1_matrix_2022", "Signal list"=w148, "Signal data"=w149) -> ("Signal"=w152:dbl)
                  n64 = call "get_signal_by_name.vi"("Signal name"=refnum<k21> "APPS1_ADC\nCAN1_matrix_2022" ("y"), "Signal list"=w148, "Signal data"=w149) -> ("Signal"=w153:dbl)
                  n65 = Bundle(cluster=T16 {"APPS1_ADC"=0.0, "APPS2_ADC"=0.0, "PPS1_ADC"=0.0, "PPS2_ADC"=0.0}, "APPS1_ADC"=w153, "APPS2_ADC"=w150, "PPS1_ADC"=w151, "PPS2_ADC"=w152) -> (→"512":T16)
                }
                frame 1409 {
                  n66 = call "get_signal_by_name.vi"("Signal name"=refnum<k21> "Pedal_Node_heartbeat\nCAN1_matrix_2022", "Signal list"=w160, "Signal data"=w161) -> ("Signal"=→"1409":dbl)
                }
                frame 81911111 {
                  n67 = call "get_signal_by_name.vi"("Signal name"=refnum<k21> "ASF_BFS_Vectornav_12V\nCAN1_matrix_2022", "Signal list"=w174, "Signal data"=w175) -> ("Signal"=w238:dbl)
                  n68 = call "get_signal_by_name.vi"("Signal name"=refnum<k21> "ASMS\nCAN1_matrix_2022", "Signal list"=w174, "Signal data"=w175) -> ("Signal"=w237:dbl)
                  n69 = call "get_signal_by_name.vi"("Signal name"=refnum<k21> "ASSI_state\nCAN1_matrix_2022", "Signal list"=w174, "Signal data"=w175) -> ("Signal"=w232:dbl)
                  n70 = call "get_signal_by_name.vi"("Signal name"=refnum<k21> "AS_GO_Signal\nCAN1_matrix_2022", "Signal list"=w174, "Signal data"=w175) -> ("Signal"=w233:dbl)
                  n71 = call "get_signal_by_name.vi"("Signal name"=refnum<k21> "AS_Mission_selected\nCAN1_matrix_2022", "Signal list"=w174, "Signal data"=w175) -> ("Signal"=w234:dbl)
                  n72 = call "get_signal_by_name.vi"("Signal name"=refnum<k21> "Brake_Light\nCAN1_matrix_2022", "Signal list"=w174, "Signal data"=w175) -> ("Signal"=w235:dbl)
                  n73 = call "get_signal_by_name.vi"("Signal name"=refnum<k21> "Buzzer\nCAN1_matrix_2022", "Signal list"=w174, "Signal data"=w175) -> ("Signal"=w236:dbl)
                  n74 = call "get_signal_by_name.vi"("Signal name"=refnum<k21> "CAN_Nodes_24V\nCAN1_matrix_2022", "Signal list"=w174, "Signal data"=w175) -> ("Signal"=w227:dbl)
                  n75 = call "get_signal_by_name.vi"("Signal name"=refnum<k21> "Calibration_Enabled\nCAN1_matrix_2022", "Signal list"=w174, "Signal data"=w175) -> ("Signal"=w226:dbl)
                  n76 = call "get_signal_by_name.vi"("Signal name"=refnum<k21> "Calibration_State\nCAN1_matrix_2022", "Signal list"=w174, "Signal data"=w175) -> ("Signal"=w225:dbl)
                  n77 = call "get_signal_by_name.vi"("Signal name"=refnum<k21> "Can_Nodes_Configured\nCAN1_matrix_2022", "Signal list"=w174, "Signal data"=w175) -> ("Signal"=w211:dbl)
                  n78 = call "get_signal_by_name.vi"("Signal name"=refnum<k21> "Datalogger_2D_12V\nCAN1_matrix_2022", "Signal list"=w174, "Signal data"=w175) -> ("Signal"=w210:dbl)
                  n79 = call "get_signal_by_name.vi"("Signal name"=refnum<k21> "Driving_State_Active\nCAN1_matrix_2022", "Signal list"=w174, "Signal data"=w175) -> ("Signal"=w209:dbl)
                  n80 = call "get_signal_by_name.vi"("Signal name"=refnum<k21> "EBS_FB\nCAN1_matrix_2022", "Signal list"=w174, "Signal data"=w175) -> ("Signal"=w208:dbl)
                  n81 = call "get_signal_by_name.vi"("Signal name"=refnum<k21> "EBS_IS_ACTIVE\nCAN1_matrix_2022", "Signal list"=w174, "Signal data"=w175) -> ("Signal"=w207:dbl)
                  n82 = call "get_signal_by_name.vi"("Signal name"=refnum<k21> "External_TS_Button\nCAN1_matrix_2022", "Signal list"=w174, "Signal data"=w175) -> ("Signal"=w205:dbl)
                  n83 = call "get_signal_by_name.vi"("Signal name"=refnum<k21> "SB_ENGAGE\nCAN1_matrix_2022", "Signal list"=w174, "Signal data"=w175) -> ("Signal"=w188:dbl)
                  n84 = call "get_signal_by_name.vi"("Signal name"=refnum<k21> "SB_FB\nCAN1_matrix_2022", "Signal list"=w174, "Signal data"=w175) -> ("Signal"=w187:dbl)
                  n85 = call "get_signal_by_name.vi"("Signal name"=refnum<k21> "MCU_EF_State\nCAN1_matrix_2022", "Signal list"=w174, "Signal data"=w175) -> ("Signal"=w198:dbl)
                  n86 = call "get_signal_by_name.vi"("Signal name"=refnum<k21> "OFF_Car_State\nCAN1_matrix_2022", "Signal list"=w174, "Signal data"=w175) -> ("Signal"=w194:dbl)
                  n87 = call "get_signal_by_name.vi"("Signal name"=refnum<k21> "ON_Car_State\nCAN1_matrix_2022", "Signal list"=w174, "Signal data"=w175) -> ("Signal"=w193:dbl)
                  n88 = call "get_signal_by_name.vi"("Signal name"=refnum<k21> "Initial_Checkup_state\nCAN1_matrix_2022", "Signal list"=w174, "Signal data"=w175) -> ("Signal"=w199:dbl)
                  n89 = call "get_signal_by_name.vi"("Signal name"=refnum<k21> "MCU_FRONT_SUPPLY\nCAN1_matrix_2022", "Signal list"=w174, "Signal data"=w175) -> ("Signal"=w197:dbl)
                  n90 = call "get_signal_by_name.vi"("Signal name"=refnum<k21> "MCU_RF_State\nCAN1_matrix_2022", "Signal list"=w174, "Signal data"=w175) -> ("Signal"=w195:dbl)
                  n91 = call "get_signal_by_name.vi"("Signal name"=refnum<k21> "PPS1\nCAN1_matrix_2022", "Signal list"=w174, "Signal data"=w175) -> ("Signal"=w192:dbl)
                  n92 = call "get_signal_by_name.vi"("Signal name"=refnum<k21> "Pump\nCAN1_matrix_2022", "Signal list"=w174, "Signal data"=w175) -> ("Signal"=w190:dbl)
                  n93 = call "get_signal_by_name.vi"("Signal name"=refnum<k21> "RTDS\nCAN1_matrix_2022", "Signal list"=w174, "Signal data"=w175) -> ("Signal"=w189:dbl)
                  n94 = call "get_signal_by_name.vi"("Signal name"=refnum<k21> "MCU_REAR_SUPPLY\nCAN1_matrix_2022", "Signal list"=w174, "Signal data"=w175) -> ("Signal"=w196:dbl)
                  n95 = call "get_signal_by_name.vi"("Signal name"=refnum<k21> "PPS2\nCAN1_matrix_2022", "Signal list"=w174, "Signal data"=w175) -> ("Signal"=w191:dbl)
                  n96 = call "get_signal_by_name.vi"("Signal name"=refnum<k21> "SC_Close\nCAN1_matrix_2022", "Signal list"=w174, "Signal data"=w175) -> ("Signal"=w173:dbl)
                  n97 = call "get_signal_by_name.vi"("Signal name"=refnum<k21> "SC_START\nCAN1_matrix_2022", "Signal list"=w174, "Signal data"=w175) -> ("Signal"=w172:dbl)
                  n98 = call "get_signal_by_name.vi"("Signal name"=refnum<k21> "SET_FINISH_STATE\nCAN1_matrix_2022", "Signal list"=w174, "Signal data"=w175) -> ("Signal"=w171:dbl)
                  n99 = call "get_signal_by_name.vi"("Signal name"=refnum<k21> "START_Car_State\nCAN1_matrix_2022", "Signal list"=w174, "Signal data"=w175) -> ("Signal"=w170:dbl)
                  n100 = call "get_signal_by_name.vi"("Signal name"=refnum<k21> "TCU_Power\nCAN1_matrix_2022", "Signal list"=w174, "Signal data"=w175) -> ("Signal"=w169:dbl)
                  n101 = call "get_signal_by_name.vi"("Signal name"=refnum<k21> "WATCHDOG\nCAN1_matrix_2022", "Signal list"=w174, "Signal data"=w175) -> ("Signal"=w168:dbl)
                  n102 = call "get_signal_by_name.vi"("Signal name"=refnum<k21> "Xavier_12V\nCAN1_matrix_2022", "Signal list"=w174, "Signal data"=w175) -> ("Signal"=w167:dbl)
                  n103 = call "get_signal_by_name.vi"("Signal name"=refnum<k21> "nEBS_ENGAGE\nCAN1_matrix_2022", "Signal list"=w174, "Signal data"=w175) -> ("Signal"=w166:dbl)
                  n104 = call "get_signal_by_name.vi"("Signal name"=refnum<k21> "nEBS_IS_TRIGGERED\nCAN1_matrix_2022", "Signal list"=w174, "Signal data"=w175) -> ("Signal"=w165:dbl)
                  n105 = call "get_signal_by_name.vi"("Signal name"=refnum<k21> "nEBS_SET_ACTIVE\nCAN1_matrix_2022", "Signal list"=w174, "Signal data"=w175) -> ("Signal"=w164:dbl)
                  n106 = call "get_signal_by_name.vi"("Signal name"=refnum<k21> "nSet_Driving_State\nCAN1_matrix_2022", "Signal list"=w174, "Signal data"=w175) -> ("Signal"=w163:dbl)
                  n107 = Bundle(cluster=T26 {"ASF_BFS_Vectornav_12V"=0.0, "ASMS"=0.0, "ASSI_state"=0.0, "AS_GO_Signal"=0.0, "AS_Mission_selected"=0.0, "Brake_Light"=0.0, "Buzzer"=0.0, "CAN_Nodes_24V"=0.0, "Calibration_Enabled"=0.0, "Calibration_State"=0.0, "Can_Nodes_Configured"=0.0, "Datalogger_2D_12V"=0.0, "Driving_State_Active"=0.0, "EBS_FB"=0.0, "EBS_IS_ACTIVE"=0.0, "External_TS_Button"=0.0, "Initial_Checkup_state"=0.0, "MCU_EF_State"=0.0, "MCU_FRONT_SUPPLY"=0.0, "MCU_REAR_SUPPLY"=0.0, "MCU_RF_State"=0.0, "OFF_Car_State"=0.0, "ON_Car_State"=0.0, "PPS1"=0.0, "PPS2"=0.0, "Pump"=0.0, "RTDS"=0.0, "SB_ENGAGE"=0.0, "SB_FB"=0.0, "SC_Close"=0.0, "SC_START"=0.0, "SET_FINISH_STATE"=0.0, "START_Car_State"=0.0, "TCU_Power"=0.0, "WATCHDOG"=0.0, "Xavier_12V"=0.0, "nEBS_ENGAGE"=0.0, "nEBS_IS_TRIGGERED"=0.0, "nEBS_SET_ACTIVE"=0.0, "nSet_Driving_State"=0.0}, "ASF_BFS_Vectornav_12V"=w238, "ASMS"=w237, "ASSI_state"=w232, "AS_GO_Signal"=w233, "AS_Mission_selected"=w234, "Brake_Light"=w235, "Buzzer"=w236, "CAN_Nodes_24V"=w227, "Calibration_Enabled"=w226, "Calibration_State"=w225, "Can_Nodes_Configured"=w211, "Datalogger_2D_12V"=w210, "Driving_State_Active"=w209, "EBS_FB"=w208, "EBS_IS_ACTIVE"=w207, "External_TS_Button"=w205, "Initial_Checkup_state"=w199, "MCU_EF_State"=w198, "MCU_FRONT_SUPPLY"=w197, "MCU_REAR_SUPPLY"=w196, "MCU_RF_State"=w195, "OFF_Car_State"=w194, "ON_Car_State"=w193, "PPS1"=w192, "PPS2"=w191, "Pump"=w190, "RTDS"=w189, "SB_ENGAGE"=w188, "SB_FB"=w187, "SC_Close"=w173, "SC_START"=w172, "SET_FINISH_STATE"=w171, "START_Car_State"=w170, "TCU_Power"=w169, "WATCHDOG"=w168, "Xavier_12V"=w167, "nEBS_ENGAGE"=w166, "nEBS_IS_TRIGGERED"=w165, "nEBS_SET_ACTIVE"=w164, "nSet_Driving_State"=w163) -> ()  [unwired: 1 out]
                }
                frame 819 {
                  n108 = call "get_signals_by_name.vi"("Signals to read"=refnum<k21>[] ["ASF_BFS_Vectornav_12V\nCAN1_matrix_2022", "ASMS\nCAN1_matrix_2022", "ASSI_state\nCAN1_matrix_2022", "AS_GO_Signal\nCAN1_matrix_2022", "AS_Mission_selected\nCAN1_matrix_2022", "ASF_BFS_Vectornav_12V\nCAN1_matrix_2022", "Buzzer\nCAN1_matrix_2022", "CAN_Nodes_24V\nCAN1_matrix_2022", "Calibration_Enabled\nCAN1_matrix_2022", "Calibration_State\nCAN1_matrix_2022", "Can_Nodes_Configured\nCAN1_matrix_2022", "Datalogger_2D_12V\nCAN1_matrix_2022", "Driving_State_Active\nCAN1_matrix_2022", "EBS_FB\nCAN1_matrix_2022", "EBS_IS_ACTIVE\nCAN1_matrix_2022", "External_TS_Button\nCAN1_matrix_2022", "Initial_Checkup_state\nCAN1_matrix_2022", "MCU_EF_State\nCAN1_matrix_2022", "MCU_FRONT_SUPPLY\nCAN1_matrix_2022", "MCU_REAR_SUPPLY\nCAN1_matrix_2022", "MCU_RF_State\nCAN1_matrix_2022", "OFF_Car_State\nCAN1_matrix_2022", "ON_Car_State\nCAN1_matrix_2022", "PPS1\nCAN1_matrix_2022", "PPS2\nCAN1_matrix_2022", "Pump\nCAN1_matrix_2022", "RTDS\nCAN1_matrix_2022", "SB_ENGAGE\nCAN1_matrix_2022", "SB_FB\nCAN1_matrix_2022", "SC_Close\nCAN1_matrix_2022", "SC_START\nCAN1_matrix_2022", "SET_FINISH_STATE\nCAN1_matrix_2022", "START_Car_State\nCAN1_matrix_2022", "TCU_Power\nCAN1_matrix_2022", "WATCHDOG\nCAN1_matrix_2022", "Xavier_12V\nCAN1_matrix_2022", "nEBS_ENGAGE\nCAN1_matrix_2022", "nEBS_IS_TRIGGERED\nCAN1_matrix_2022", "nEBS_SET_ACTIVE\nCAN1_matrix_2022", "nSet_Driving_State\nCAN1_matrix_2022"], "Signal list"=w248, "Signal data"=w247) -> ("Signals"=→"819":dbl[])
                }
                frame 820 {
                  n109 = call "get_signal_by_name.vi"("Signal name"=refnum<k21> "ACCELERATION_LED\nCAN1_matrix_2022", "Signal list"=w254, "Signal data"=w255) -> ("Signal"=w310:dbl)
                  n110 = call "get_signal_by_name.vi"("Signal name"=refnum<k21> "AMS_LED\nCAN1_matrix_2022", "Signal list"=w254, "Signal data"=w255) -> ("Signal"=w309:dbl)
                  n111 = call "get_signal_by_name.vi"("Signal name"=refnum<k21> "ASB_ERROR_LED\nCAN1_matrix_2022", "Signal list"=w254, "Signal data"=w255) -> ("Signal"=w304:dbl)
                  n112 = call "get_signal_by_name.vi"("Signal name"=refnum<k21> "AUTOX_LED\nCAN1_matrix_2022", "Signal list"=w254, "Signal data"=w255) -> ("Signal"=w305:dbl)
                  n113 = call "get_signal_by_name.vi"("Signal name"=refnum<k21> "Dashboard_heartbeat_error\nCAN1_matrix_2022", "Signal list"=w254, "Signal data"=w255) -> ("Signal"=w306:dbl)
                  n114 = call "get_signal_by_name.vi"("Signal name"=refnum<k21> "EBS_TEST_LED\nCAN1_matrix_2022", "Signal list"=w254, "Signal data"=w255) -> ("Signal"=w307:dbl)
                  n115 = call "get_signal_by_name.vi"("Signal name"=refnum<k21> "HVECU_Heartbeat_error\nCAN1_matrix_2022", "Signal list"=w254, "Signal data"=w255) -> ("Signal"=w308:dbl)
                  n116 = call "get_signal_by_name.vi"("Signal name"=refnum<k21> "HV_LED\nCAN1_matrix_2022", "Signal list"=w254, "Signal data"=w255) -> ("Signal"=w299:dbl)
                  n117 = call "get_signal_by_name.vi"("Signal name"=refnum<k21> "IMD_LED\nCAN1_matrix_2022", "Signal list"=w254, "Signal data"=w255) -> ("Signal"=w298:dbl)
                  n118 = call "get_signal_by_name.vi"("Signal name"=refnum<k21> "INSPECTION_LED\nCAN1_matrix_2022", "Signal list"=w254, "Signal data"=w255) -> ("Signal"=w297:dbl)
                  n119 = call "get_signal_by_name.vi"("Signal name"=refnum<k21> "MANUAL_MODE_LED\nCAN1_matrix_2022", "Signal list"=w254, "Signal data"=w255) -> ("Signal"=w283:dbl)
                  n120 = call "get_signal_by_name.vi"("Signal name"=refnum<k21> "MCU1_LED\nCAN1_matrix_2022", "Signal list"=w254, "Signal data"=w255) -> ("Signal"=w282:dbl)
                  n121 = call "get_signal_by_name.vi"("Signal name"=refnum<k21> "MCU2_LED\nCAN1_matrix_2022", "Signal list"=w254, "Signal data"=w255) -> ("Signal"=w281:dbl)
                  n122 = call "get_signal_by_name.vi"("Signal name"=refnum<k21> "MCU3_LED\nCAN1_matrix_2022", "Signal list"=w254, "Signal data"=w255) -> ("Signal"=w280:dbl)
                  n123 = call "get_signal_by_name.vi"("Signal name"=refnum<k21> "MCU4_LED\nCAN1_matrix_2022", "Signal list"=w254, "Signal data"=w255) -> ("Signal"=w279:dbl)
                  n124 = call "get_signal_by_name.vi"("Signal name"=refnum<k21> "MCU_Heartbeat_error\nCAN1_matrix_2022", "Signal list"=w254, "Signal data"=w255) -> ("Signal"=w277:dbl)
                  n125 = call "get_signal_by_name.vi"("Signal name"=refnum<k21> "Steering_Heartbeat_error\nCAN1_matrix_2022", "Signal list"=w254, "Signal data"=w255) -> ("Signal"=w260:dbl)
                  n126 = call "get_signal_by_name.vi"("Signal name"=refnum<k21> "TCU_Heartbeat_error\nCAN1_matrix_2022", "Signal list"=w254, "Signal data"=w255) -> ("Signal"=w259:dbl)
                  n127 = call "get_signal_by_name.vi"("Signal name"=refnum<k21> "SC_BSPD_FB\nCAN1_matrix_2022", "Signal list"=w254, "Signal data"=w255) -> ("Signal"=w270:dbl)
                  n128 = call "get_signal_by_name.vi"("Signal name"=refnum<k21> "SC_ENDLINE_ADC\nCAN1_matrix_2022", "Signal list"=w254, "Signal data"=w255) -> ("Signal"=w266:dbl)
                  n129 = call "get_signal_by_name.vi"("Signal name"=refnum<k21> "SC_FRONT_FB\nCAN1_matrix_2022", "Signal list"=w254, "Signal data"=w255) -> ("Signal"=w265:dbl)
                  n130 = call "get_signal_by_name.vi"("Signal name"=refnum<k21> "Pedal_Node_Heartbeat_error\nCAN1_matrix_2022", "Signal list"=w254, "Signal data"=w255) -> ("Signal"=w271:dbl)
                  n131 = call "get_signal_by_name.vi"("Signal name"=refnum<k21> "SC_DV_FB\nCAN1_matrix_2022", "Signal list"=w254, "Signal data"=w255) -> ("Signal"=w269:dbl)
                  n132 = call "get_signal_by_name.vi"("Signal name"=refnum<k21> "SC_EBS_FB\nCAN1_matrix_2022", "Signal list"=w254, "Signal data"=w255) -> ("Signal"=w267:dbl)
                  n133 = call "get_signal_by_name.vi"("Signal name"=refnum<k21> "SC_HOOP_FB\nCAN1_matrix_2022", "Signal list"=w254, "Signal data"=w255) -> ("Signal"=w264:dbl)
                  n134 = call "get_signal_by_name.vi"("Signal name"=refnum<k21> "SKIDPAD_LED\nCAN1_matrix_2022", "Signal list"=w254, "Signal data"=w255) -> ("Signal"=w262:dbl)
                  n135 = call "get_signal_by_name.vi"("Signal name"=refnum<k21> "SSG_Heartbeat\nCAN1_matrix_2022", "Signal list"=w254, "Signal data"=w255) -> ("Signal"=w261:dbl)
                  n136 = call "get_signal_by_name.vi"("Signal name"=refnum<k21> "SC_DV_RELAY_FB\nCAN1_matrix_2022", "Signal list"=w254, "Signal data"=w255) -> ("Signal"=w268:dbl)
                  n137 = call "get_signal_by_name.vi"("Signal name"=refnum<k21> "SC_MCU_FB\nCAN1_matrix_2022", "Signal list"=w254, "Signal data"=w255) -> ("Signal"=w263:dbl)
                  n138 = call "get_signal_by_name.vi"("Signal name"=refnum<k21> "TCU_LED\nCAN1_matrix_2022", "Signal list"=w254, "Signal data"=w255) -> ("Signal"=w253:dbl)
                  n139 = call "get_signal_by_name.vi"("Signal name"=refnum<k21> "TRACKDRIVE_LED\nCAN1_matrix_2022", "Signal list"=w254, "Signal data"=w255) -> ("Signal"=w252:dbl)
                  n140 = call "get_signal_by_name.vi"("Signal name"=refnum<k21> "TS_OFF_LED\nCAN1_matrix_2022", "Signal list"=w254, "Signal data"=w255) -> ("Signal"=w251:dbl)
                  n141 = Bundle(cluster=T15 {"ACCELERATION_LED"=0.0, "AMS_LED"=0.0, "ASB_ERROR_LED"=0.0, "AUTOX_LED"=0.0, "Dashboard_heartbeat_error"=0.0, "EBS_TEST_LED"=0.0, "HVECU_Heartbeat_error"=0.0, "HV_LED"=0.0, "IMD_LED"=0.0, "INSPECTION_LED"=0.0, "MANUAL_MODE_LED"=0.0, "MCU1_LED"=0.0, "MCU2_LED"=0.0, "MCU3_LED"=0.0, "MCU4_LED"=0.0, "MCU_Heartbeat_error"=0.0, "Pedal_Node_Heartbeat_error"=0.0, "SC_BSPD_FB"=0.0, "SC_DV_FB"=0.0, "SC_DV_RELAY_FB"=0.0, "SC_EBS_FB"=0.0, "SC_ENDLINE_ADC"=0.0, "SC_FRONT_FB"=0.0, "SC_HOOP_FB"=0.0, "SC_MCU_FB"=0.0, "SKIDPAD_LED"=0.0, "SSG_Heartbeat"=0.0, "Steering_Heartbeat_error"=0.0, "TCU_Heartbeat_error"=0.0, "TCU_LED"=0.0, "TRACKDRIVE_LED"=0.0, "TS_OFF_LED"=0.0}, "ACCELERATION_LED"=w310, "AMS_LED"=w309, "ASB_ERROR_LED"=w304, "AUTOX_LED"=w305, "Dashboard_heartbeat_error"=w306, "EBS_TEST_LED"=w307, "HVECU_Heartbeat_error"=w308, "HV_LED"=w299, "IMD_LED"=w298, "INSPECTION_LED"=w297, "MANUAL_MODE_LED"=w283, "MCU1_LED"=w282, "MCU2_LED"=w281, "MCU3_LED"=w280, "MCU4_LED"=w279, "MCU_Heartbeat_error"=w277, "Pedal_Node_Heartbeat_error"=w271, "SC_BSPD_FB"=w270, "SC_DV_FB"=w269, "SC_DV_RELAY_FB"=w268, "SC_EBS_FB"=w267, "SC_ENDLINE_ADC"=w266, "SC_FRONT_FB"=w265, "SC_HOOP_FB"=w264, "SC_MCU_FB"=w263, "SKIDPAD_LED"=w262, "SSG_Heartbeat"=w261, "Steering_Heartbeat_error"=w260, "TCU_Heartbeat_error"=w259, "TCU_LED"=w253, "TRACKDRIVE_LED"=w252, "TS_OFF_LED"=w251) -> (→"820":T15)
                }
                frame 873 {
                  n142 = call "get_signal_by_name.vi"("Signal name"=refnum<k21> "Steering_letter3\nCAN1_matrix_2022", "Signal list"=w320, "Signal data"=w321) -> ("Signal"=w325:dbl)
                  n143 = call "get_signal_by_name.vi"("Signal name"=refnum<k21> "Steering_number\nCAN1_matrix_2022", "Signal list"=w320, "Signal data"=w321) -> ("Signal"=w319:dbl)
                  n144 = call "get_signal_by_name.vi"("Signal name"=refnum<k21> "Steering_letter2\nCAN1_matrix_2022", "Signal list"=w320, "Signal data"=w321) -> ("Signal"=w324:dbl)
                  n145 = call "get_signal_by_name.vi"("Signal name"=refnum<k21> "Steering_letter4\nCAN1_matrix_2022", "Signal list"=w320, "Signal data"=w321) -> ("Signal"=w326:dbl)
                  n146 = call "get_signal_by_name.vi"("Signal name"=refnum<k21> "Steering_letter1\nCAN1_matrix_2022" ("y"), "Signal list"=w320, "Signal data"=w321) -> ("Signal"=w327:dbl)
                  n147 = Bundle(cluster=T14 {"Steering_letter1"=0.0, "Steering_letter2"=0.0, "Steering_letter3"=0.0, "Steering_letter4"=0.0, "Steering_number"=0.0}, "Steering_letter1"=w327, "Steering_letter2"=w324, "Steering_letter3"=w325, "Steering_letter4"=w326, "Steering_number"=w319) -> (→"873":T14)
                }
                frame 1030 {
                  n148 = call "get_signal_by_name.vi"("Signal name"=refnum<k21> "EEPROM_STA2_MAX\nCAN1_matrix_2022", "Signal list"=w333, "Signal data"=w334) -> ("Signal"=w336:dbl)
                  n149 = call "get_signal_by_name.vi"("Signal name"=refnum<k21> "EEPROM_STA1_MIN\nCAN1_matrix_2022", "Signal list"=w333, "Signal data"=w334) -> ("Signal"=w335:dbl)
                  n150 = call "get_signal_by_name.vi"("Signal name"=refnum<k21> "EEPROM_STA2_MIN\nCAN1_matrix_2022", "Signal list"=w333, "Signal data"=w334) -> ("Signal"=w337:dbl)
                  n151 = call "get_signal_by_name.vi"("Signal name"=refnum<k21> "EEPROM_STA1_MAX\nCAN1_matrix_2022" ("y"), "Signal list"=w333, "Signal data"=w334) -> ("Signal"=w338:dbl)
                  n152 = Bundle(cluster=T13 {"EEPROM_STA1_MAX"=0.0, "EEPROM_STA1_MIN"=0.0, "EEPROM_STA2_MAX"=0.0, "EEPROM_STA2_MIN"=0.0}, "EEPROM_STA1_MAX"=w338, "EEPROM_STA1_MIN"=w335, "EEPROM_STA2_MAX"=w336, "EEPROM_STA2_MIN"=w337) -> (→"1030":T13)
                }
                frame 656 {
                  n153 = call "get_signal_by_name.vi"("Signal name"=refnum<k21> "Button1\nCAN1_matrix_2022", "Signal list"=w347, "Signal data"=w348) -> ("Signal"=w358:dbl)
                  n154 = call "get_signal_by_name.vi"("Signal name"=refnum<k21> "Button2\nCAN1_matrix_2022", "Signal list"=w347, "Signal data"=w348) -> ("Signal"=w357:dbl)
                  n155 = call "get_signal_by_name.vi"("Signal name"=refnum<k21> "Button3\nCAN1_matrix_2022", "Signal list"=w347, "Signal data"=w348) -> ("Signal"=w352:dbl)
                  n156 = call "get_signal_by_name.vi"("Signal name"=refnum<k21> "Button4\nCAN1_matrix_2022", "Signal list"=w347, "Signal data"=w348) -> ("Signal"=w353:dbl)
                  n157 = call "get_signal_by_name.vi"("Signal name"=refnum<k21> "Rotary1\nCAN1_matrix_2022", "Signal list"=w347, "Signal data"=w348) -> ("Signal"=w354:dbl)
                  n158 = call "get_signal_by_name.vi"("Signal name"=refnum<k21> "Rotary3\nCAN1_matrix_2022", "Signal list"=w347, "Signal data"=w348) -> ("Signal"=w356:dbl)
                  n159 = call "get_signal_by_name.vi"("Signal name"=refnum<k21> "Rotary4\nCAN1_matrix_2022", "Signal list"=w347, "Signal data"=w348) -> ("Signal"=w346:dbl)
                  n160 = call "get_signal_by_name.vi"("Signal name"=refnum<k21> "Steering_heartbeat\nCAN1_matrix_2022", "Signal list"=w347, "Signal data"=w348) -> ("Signal"=w344:dbl)
                  n161 = call "get_signal_by_name.vi"("Signal name"=refnum<k21> "Rotary2\nCAN1_matrix_2022", "Signal list"=w347, "Signal data"=w348) -> ("Signal"=w355:dbl)
                  n162 = call "get_signal_by_name.vi"("Signal name"=refnum<k21> "Rotary5\nCAN1_matrix_2022", "Signal list"=w347, "Signal data"=w348) -> ("Signal"=w345:dbl)
                  n163 = Bundle(cluster=T27 {"Button1"=0.0, "Button2"=0.0, "Button3"=0.0, "Button4"=0.0, "Rotary1"=0.0, "Rotary2"=0.0, "Rotary3"=0.0, "Rotary4"=0.0, "Rotary5"=0.0, "Steering_heartbeat"=0.0}, "Button1"=w358, "Button2"=w357, "Button3"=w352, "Button4"=w353, "Rotary1"=w354, "Rotary2"=w355, "Rotary3"=w356, "Rotary4"=w346, "Rotary5"=w345, "Steering_heartbeat"=w344) -> ()  [unwired: 1 out]
                }
                frame 1153 {
                  n164 = call "get_signal_by_name.vi"("Signal name"=refnum<k21> "VDC_Brake_Force_Max\nCAN1_matrix_2022", "Signal list"=w369, "Signal data"=w370) -> ("Signal"=w385:dbl)
                  n165 = call "get_signal_by_name.vi"("Signal name"=refnum<k21> "VDC_Brake_Force_Threshold\nCAN1_matrix_2022", "Signal list"=w369, "Signal data"=w370) -> ("Signal"=w384:dbl)
                  n166 = call "get_signal_by_name.vi"("Signal name"=refnum<k21> "VDC_Drop_Parameter_New\nCAN1_matrix_2022", "Signal list"=w369, "Signal data"=w370) -> ("Signal"=w379:dbl)
                  n167 = call "get_signal_by_name.vi"("Signal name"=refnum<k21> "VDC_M_Yaw\nCAN1_matrix_2022", "Signal list"=w369, "Signal data"=w370) -> ("Signal"=w380:dbl)
                  n168 = call "get_signal_by_name.vi"("Signal name"=refnum<k21> "VDC_M_Yaw_Limit\nCAN1_matrix_2022", "Signal list"=w369, "Signal data"=w370) -> ("Signal"=w381:dbl)
                  n169 = call "get_signal_by_name.vi"("Signal name"=refnum<k21> "VDC_Powlim_Approx\nCAN1_matrix_2022", "Signal list"=w369, "Signal data"=w370) -> ("Signal"=w382:dbl)
                  n170 = call "get_signal_by_name.vi"("Signal name"=refnum<k21> "VDC_Rear_Reduction\nCAN1_matrix_2022", "Signal list"=w369, "Signal data"=w370) -> ("Signal"=w383:dbl)
                  n171 = call "get_signal_by_name.vi"("Signal name"=refnum<k21> "VDC_TC_Normalizer\nCAN1_matrix_2022", "Signal list"=w369, "Signal data"=w370) -> ("Signal"=w375:dbl)
                  n172 = call "get_signal_by_name.vi"("Signal name"=refnum<k21> "VDC_Throttle_Bias\nCAN1_matrix_2022", "Signal list"=w369, "Signal data"=w370) -> ("Signal"=w374:dbl)
                  n173 = call "get_signal_by_name.vi"("Signal name"=refnum<k21> "VDC_Yaw_Control_Balance\nCAN1_matrix_2022", "Signal list"=w369, "Signal data"=w370) -> ("Signal"=w373:dbl)
                  n174 = call "get_signal_by_name.vi"("Signal name"=refnum<k21> "VDC_Yaw_Control_Weight_Selector\nCAN1_matrix_2022", "Signal list"=w369, "Signal data"=w370) -> ("Signal"=w368:dbl)
                  n175 = Bundle(cluster=T12 {"VDC_Brake_Force_Max"=0.0, "VDC_Brake_Force_Threshold"=0.0, "VDC_Drop_Parameter_New"=0.0, "VDC_M_Yaw"=0.0, "VDC_M_Yaw_Limit"=0.0, "VDC_Powlim_Approx"=0.0, "VDC_Rear_Reduction"=0.0, "VDC_TC_Normalizer"=0.0, "VDC_Throttle_Bias"=0.0, "VDC_Yaw_Control_Balance"=0.0, "VDC_Yaw_Control_Weight_Selector"=0.0}, "VDC_Brake_Force_Max"=w385, "VDC_Brake_Force_Threshold"=w384, "VDC_Drop_Parameter_New"=w379, "VDC_M_Yaw"=w380, "VDC_M_Yaw_Limit"=w381, "VDC_Powlim_Approx"=w382, "VDC_Rear_Reduction"=w383, "VDC_TC_Normalizer"=w375, "VDC_Throttle_Bias"=w374, "VDC_Yaw_Control_Balance"=w373, "VDC_Yaw_Control_Weight_Selector"=w368) -> (→"1153":T12)
                }
                frame 1157 {
                  n176 = call "get_signal_by_name.vi"("Signal name"=refnum<k21> "VDC_Fz_FL\nCAN1_matrix_2022", "Signal list"=w394, "Signal data"=w395) -> ("Signal"=w405:dbl)
                  n177 = call "get_signal_by_name.vi"("Signal name"=refnum<k21> "VDC_Fz_FR\nCAN1_matrix_2022", "Signal list"=w394, "Signal data"=w395) -> ("Signal"=w404:dbl)
                  n178 = call "get_signal_by_name.vi"("Signal name"=refnum<k21> "VDC_Fz_RL\nCAN1_matrix_2022", "Signal list"=w394, "Signal data"=w395) -> ("Signal"=w399:dbl)
                  n179 = call "get_signal_by_name.vi"("Signal name"=refnum<k21> "VDC_Fz_RR\nCAN1_matrix_2022", "Signal list"=w394, "Signal data"=w395) -> ("Signal"=w400:dbl)
                  n180 = call "get_signal_by_name.vi"("Signal name"=refnum<k21> "VDC_Regbrake_Front\nCAN1_matrix_2022", "Signal list"=w394, "Signal data"=w395) -> ("Signal"=w401:dbl)
                  n181 = call "get_signal_by_name.vi"("Signal name"=refnum<k21> "VDC_Regbrake_Rear\nCAN1_matrix_2022", "Signal list"=w394, "Signal data"=w395) -> ("Signal"=w402:dbl)
                  n182 = call "get_signal_by_name.vi"("Signal name"=refnum<k21> "VDC_Torque_Demand\nCAN1_matrix_2022", "Signal list"=w394, "Signal data"=w395) -> ("Signal"=w403:dbl)
                  n183 = call "get_signal_by_name.vi"("Signal name"=refnum<k21> "VDC_v_x\nCAN1_matrix_2022", "Signal list"=w394, "Signal data"=w395) -> ("Signal"=w397:dbl)
                  n184 = Bundle(cluster=T11 {"VDC_Fz_FL"=0.0, "VDC_Fz_FR"=0.0, "VDC_Fz_RL"=0.0, "VDC_Fz_RR"=0.0, "VDC_Regbrake_Front"=0.0, "VDC_Regbrake_Rear"=0.0, "VDC_Torque_Demand"=0.0, "VDC_v_x"=0.0}, "VDC_Fz_FL"=w405, "VDC_Fz_FR"=w404, "VDC_Fz_RL"=w399, "VDC_Fz_RR"=w400, "VDC_Regbrake_Front"=w401, "VDC_Regbrake_Rear"=w402, "VDC_Torque_Demand"=w403, "VDC_v_x"=w397) -> (→"1157":T11)
                }
                frame 1029 {
                  n185 = call "get_signal_by_name.vi"("Signal name"=refnum<k21> "EEPROM_APPS1_MAX\nCAN1_matrix_2022", "Signal list"=w414, "Signal data"=w415) -> ("Signal"=w420:dbl)
                  n186 = call "get_signal_by_name.vi"("Signal name"=refnum<k21> "EEPROM_APPS1_MIN\nCAN1_matrix_2022", "Signal list"=w414, "Signal data"=w415) -> ("Signal"=w419:dbl)
                  n187 = call "get_signal_by_name.vi"("Signal name"=refnum<k21> "EEPROM_APPS2_MAX\nCAN1_matrix_2022", "Signal list"=w414, "Signal data"=w415) -> ("Signal"=w417:dbl)
                  n188 = call "get_signal_by_name.vi"("Signal name"=refnum<k21> "EEPROM_APPS2_MIN\nCAN1_matrix_2022", "Signal list"=w414, "Signal data"=w415) -> ("Signal"=w418:dbl)
                  n189 = Bundle(cluster=T10 {"EEPROM_APPS1_MAX"=0.0, "EEPROM_APPS1_MIN"=0.0, "EEPROM_APPS2_MAX"=0.0, "EEPROM_APPS2_MIN"=0.0}, "EEPROM_APPS1_MAX"=w420, "EEPROM_APPS1_MIN"=w419, "EEPROM_APPS2_MAX"=w417, "EEPROM_APPS2_MIN"=w418) -> (→"1029":T10)
                }
                frame 560 {
                  n190 = call "get_signal_by_name.vi"("Signal name"=refnum<k21> "APPS1_position\nCAN1_matrix_2022", "Signal list"=w425, "Signal data"=w426) -> ("Signal"=w439:dbl)
                  n191 = call "get_signal_by_name.vi"("Signal name"=refnum<k21> "APPS1_validity\nCAN1_matrix_2022", "Signal list"=w425, "Signal data"=w426) -> ("Signal"=w438:dbl)
                  n192 = call "get_signal_by_name.vi"("Signal name"=refnum<k21> "APPS2_posiition\nCAN1_matrix_2022", "Signal list"=w425, "Signal data"=w426) -> ("Signal"=w433:dbl)
                  n193 = call "get_signal_by_name.vi"("Signal name"=refnum<k21> "APPS2_validity\nCAN1_matrix_2022", "Signal list"=w425, "Signal data"=w426) -> ("Signal"=w434:dbl)
                  n194 = call "get_signal_by_name.vi"("Signal name"=refnum<k21> "APPS_plausiblity\nCAN1_matrix_2022", "Signal list"=w425, "Signal data"=w426) -> ("Signal"=w435:dbl)
                  n195 = call "get_signal_by_name.vi"("Signal name"=refnum<k21> "STA1_validity\nCAN1_matrix_2022", "Signal list"=w425, "Signal data"=w426) -> ("Signal"=w437:dbl)
                  n196 = call "get_signal_by_name.vi"("Signal name"=refnum<k21> "STA2_position\nCAN1_matrix_2022", "Signal list"=w425, "Signal data"=w426) -> ("Signal"=w429:dbl)
                  n197 = call "get_signal_by_name.vi"("Signal name"=refnum<k21> "STA_plausiblity\nCAN1_matrix_2022", "Signal list"=w425, "Signal data"=w426) -> ("Signal"=w427:dbl)
                  n198 = call "get_signal_by_name.vi"("Signal name"=refnum<k21> "STA1_position\nCAN1_matrix_2022", "Signal list"=w425, "Signal data"=w426) -> ("Signal"=w436:dbl)
                  n199 = call "get_signal_by_name.vi"("Signal name"=refnum<k21> "STA2_validity\nCAN1_matrix_2022", "Signal list"=w425, "Signal data"=w426) -> ("Signal"=w428:dbl)
                  n200 = Bundle(cluster=T28 {"APPS1_position"=0.0, "APPS1_validity"=0.0, "APPS2_posiition"=0.0, "APPS2_validity"=0.0, "APPS_plausiblity"=0.0, "STA1_position"=0.0, "STA1_validity"=0.0, "STA2_position"=0.0, "STA2_validity"=0.0, "STA_plausiblity"=0.0}, "APPS1_position"=w439, "APPS1_validity"=w438, "APPS2_posiition"=w433, "APPS2_validity"=w434, "APPS_plausiblity"=w435, "STA1_position"=w436, "STA1_validity"=w437, "STA2_position"=w429, "STA2_validity"=w428, "STA_plausiblity"=w427) -> ()  [unwired: 1 out]
                }
                frame 105 {
                  n201 = call "get_signal_by_name.vi"("Signal name"=refnum<k21> "Xavier_Target_speed\nCAN1_matrix_2022", "Signal list"=w450, "Signal data"=w449) -> ("Signal"=w452:dbl)
                  n202 = call "get_signal_by_name.vi"("Signal name"=refnum<k21> "Xavier_Target_Steering_Angle\nCAN1_matrix_2022", "Signal list"=w450, "Signal data"=w449) -> ("Signal"=w451:dbl)
                  n203 = call "get_signal_by_name.vi"("Signal name"=refnum<k21> "Xavier_heartbeat\nCAN1_matrix_2022", "Signal list"=w450, "Signal data"=w449) -> ("Signal"=w453:dbl)
                  n204 = call "get_signal_by_name.vi"("Signal name"=refnum<k21> "Xavier_AS_Finish\nCAN1_matrix_2022" ("y"), "Signal list"=w450, "Signal data"=w449) -> ("Signal"=w454:dbl)
                  n205 = Bundle(cluster=T9 {"Xavier_AS_Finish"=0.0, "Xavier_Target_Steering_Angle"=0.0, "Xavier_Target_speed"=0.0, "Xavier_heartbeat"=0.0}, "Xavier_AS_Finish"=w454, "Xavier_Target_Steering_Angle"=w451, "Xavier_Target_speed"=w452, "Xavier_heartbeat"=w453) -> (→"105":T9)
                }
                frame 648 {
                  n206 = call "get_signal_by_name.vi"("Signal name"=refnum<k21> "AMK3_status\nCAN2_matrix_2022", "Signal list"=w465, "Signal data"=w466) -> ("Signal"=w468:dbl)
                  n207 = call "get_signal_by_name.vi"("Signal name"=refnum<k21> "AMK3_torque_current\nCAN2_matrix_2022", "Signal list"=w465, "Signal data"=w466) -> ("Signal"=w469:dbl)
                  n208 = call "get_signal_by_name.vi"("Signal name"=refnum<k21> "AMK3_actual_velocity\nCAN2_matrix_2022", "Signal list"=w465, "Signal data"=w466) -> ("Signal"=w470:dbl)
                  n209 = call "get_signal_by_name.vi"("Signal name"=refnum<k21> "AMK3_magnetizing_current\nCAN2_matrix_2022", "Signal list"=w465, "Signal data"=w466) -> ("Signal"=w467:dbl)
                  n210 = Bundle(cluster=T8 {"AMK3_actual_velocitiy"=0.0, "AMK3_magnetizing_current"=0.0, "AMK3_status"=0.0, "AMK3_torque_current"=0.0}, "AMK3_actual_velocitiy"=w470, "AMK3_magnetizing_current"=w467, "AMK3_status"=w468, "AMK3_torque_current"=w469) -> (→"648":T8)
                }
                frame 649 {
                  n211 = call "get_signal_by_name.vi"("Signal name"=refnum<k21> "AMK4_status\nCAN2_matrix_2022", "Signal list"=w477, "Signal data"=w478) -> ("Signal"=w480:dbl)
                  n212 = call "get_signal_by_name.vi"("Signal name"=refnum<k21> "AMK4_torque_current\nCAN2_matrix_2022", "Signal list"=w477, "Signal data"=w478) -> ("Signal"=w481:dbl)
                  n213 = call "get_signal_by_name.vi"("Signal name"=refnum<k21> "AMK4_actual_velocity\nCAN2_matrix_2022", "Signal list"=w477, "Signal data"=w478) -> ("Signal"=w482:dbl)
                  n214 = call "get_signal_by_name.vi"("Signal name"=refnum<k21> "AMK4_magnetizing_current\nCAN2_matrix_2022", "Signal list"=w477, "Signal data"=w478) -> ("Signal"=w479:dbl)
                  n215 = Bundle(cluster=T7 {"AMK4_actual_velocitiy"=0.0, "AMK4_magnetizing_current"=0.0, "AMK4_status"=0.0, "AMK4_torque_current"=0.0}, "AMK4_actual_velocitiy"=w482, "AMK4_magnetizing_current"=w479, "AMK4_status"=w480, "AMK4_torque_current"=w481) -> (→"649":T7)
                }
                frame 650 {
                  n216 = call "get_signal_by_name.vi"("Signal name"=refnum<k21> "AMK3_temp_inverter\nCAN2_matrix_2022", "Signal list"=w489, "Signal data"=w490) -> ("Signal"=w492:dbl)
                  n217 = call "get_signal_by_name.vi"("Signal name"=refnum<k21> "AMK3_temp_motor\nCAN2_matrix_2022", "Signal list"=w489, "Signal data"=w490) -> ("Signal"=w493:dbl)
                  n218 = call "get_signal_by_name.vi"("Signal name"=refnum<k21> "AMK3_error_info\nCAN2_matrix_2022", "Signal list"=w489, "Signal data"=w490) -> ("Signal"=w494:dbl)
                  n219 = call "get_signal_by_name.vi"("Signal name"=refnum<k21> "AMK3_temp_IGBT\nCAN2_matrix_2022", "Signal list"=w489, "Signal data"=w490) -> ("Signal"=w491:dbl)
                  n220 = Bundle(cluster=T6 {"AMK3_error_info"=0.0, "AMK3_temp_IGBT"=0.0, "AMK3_temp_inverter"=0.0, "AMK3_temp_motor"=0.0}, "AMK3_error_info"=w494, "AMK3_temp_IGBT"=w491, "AMK3_temp_inverter"=w492, "AMK3_temp_motor"=w493) -> (→"650":T6)
                }
                frame 651 {
                  n221 = call "get_signal_by_name.vi"("Signal name"=refnum<k21> "AMK4_temp_inverter\nCAN2_matrix_2022", "Signal list"=w501, "Signal data"=w502) -> ("Signal"=w504:dbl)
                  n222 = call "get_signal_by_name.vi"("Signal name"=refnum<k21> "AMK4_temp_motor\nCAN2_matrix_2022", "Signal list"=w501, "Signal data"=w502) -> ("Signal"=w505:dbl)
                  n223 = call "get_signal_by_name.vi"("Signal name"=refnum<k21> "AMK4_error_info\nCAN2_matrix_2022", "Signal list"=w501, "Signal data"=w502) -> ("Signal"=w506:dbl)
                  n224 = call "get_signal_by_name.vi"("Signal name"=refnum<k21> "AMK4_temp_IGBT\nCAN2_matrix_2022", "Signal list"=w501, "Signal data"=w502) -> ("Signal"=w503:dbl)
                  n225 = Bundle(cluster=T5 {"AMK4_error_info"=0.0, "AMK4_temp_IGBT"=0.0, "AMK4_temp_inverter"=0.0, "AMK4_temp_motor"=0.0}, "AMK4_error_info"=w506, "AMK4_temp_IGBT"=w503, "AMK4_temp_inverter"=w504, "AMK4_temp_motor"=w505) -> (→"651":T5)
                }
                frame 1378 {
                  n226 = call "get_signal_by_name.vi"("Signal name"=refnum<k21> "Button_OFF\nCAN2_matrix_2022", "Signal list"=w516, "Signal data"=w517) -> ("Signal"=w526:dbl)
                  n227 = call "get_signal_by_name.vi"("Signal name"=refnum<k21> "Button_ON\nCAN2_matrix_2022", "Signal list"=w516, "Signal data"=w517) -> ("Signal"=w525:dbl)
                  n228 = call "get_signal_by_name.vi"("Signal name"=refnum<k21> "Button_START\nCAN2_matrix_2022", "Signal list"=w516, "Signal data"=w517) -> ("Signal"=w520:dbl)
                  n229 = call "get_signal_by_name.vi"("Signal name"=refnum<k21> "Dash_BLANK\nCAN2_matrix_2022", "Signal list"=w516, "Signal data"=w517) -> ("Signal"=w521:dbl)
                  n230 = call "get_signal_by_name.vi"("Signal name"=refnum<k21> "Dash_MODE\nCAN2_matrix_2022", "Signal list"=w516, "Signal data"=w517) -> ("Signal"=w522:dbl)
                  n231 = call "get_signal_by_name.vi"("Signal name"=refnum<k21> "Dash_XLAT\nCAN2_matrix_2022", "Signal list"=w516, "Signal data"=w517) -> ("Signal"=w523:dbl)
                  n232 = call "get_signal_by_name.vi"("Signal name"=refnum<k21> "Dashboard_ID\nCAN2_matrix_2022", "Signal list"=w516, "Signal data"=w517) -> ("Signal"=w524:dbl)
                  n233 = call "get_signal_by_name.vi"("Signal name"=refnum<k21> "Dashboarrd_heartbeat\nCAN2_matrix_2022", "Signal list"=w516, "Signal data"=w517) -> ("Signal"=w519:dbl)
                  n234 = Bundle(cluster=T29 {"Button_OFF"=0.0, "Button_ON"=0.0, "Button_START"=0.0, "Dash_BLANK"=0.0, "Dash_MODE"=0.0, "Dash_XLAT"=0.0, "Dashboard_ID"=0.0, "Dashboarrd_heartbeat"=0.0}, "Button_OFF"=w526, "Button_ON"=w525, "Button_START"=w520, "Dash_BLANK"=w521, "Dash_MODE"=w522, "Dash_XLAT"=w523, "Dashboard_ID"=w524, "Dashboarrd_heartbeat"=w519) -> ()  [unwired: 1 out]
                }
                frame 530 {
                  n235 = call "get_signal_by_name.vi"("Signal name"=refnum<k21> "AIR_minus_state\nCAN2_matrix_2022", "Signal list"=w541, "Signal data"=w540) -> ("Signal"=w571:dbl)
                  n236 = call "get_signal_by_name.vi"("Signal name"=refnum<k21> "AIR_plus_State\nCAN2_matrix_2022", "Signal list"=w541, "Signal data"=w540) -> ("Signal"=w572:dbl)
                  n237 = call "get_signal_by_name.vi"("Signal name"=refnum<k21> "AMS_Relay_State\nCAN2_matrix_2022", "Signal list"=w541, "Signal data"=w540) -> ("Signal"=w577:dbl)
                  n238 = call "get_signal_by_name.vi"("Signal name"=refnum<k21> "AMS_Status\nCAN2_matrix_2022", "Signal list"=w541, "Signal data"=w540) -> ("Signal"=w576:dbl)
                  n239 = call "get_signal_by_name.vi"("Signal name"=refnum<k21> "Driver_Protection_State\nCAN2_matrix_2022", "Signal list"=w541, "Signal data"=w540) -> ("Signal"=w575:dbl)
                  n240 = call "get_signal_by_name.vi"("Signal name"=refnum<k21> "Error_STAMP_TSAL\nCAN2_matrix_2022", "Signal list"=w541, "Signal data"=w540) -> ("Signal"=w574:dbl)
                  n241 = call "get_signal_by_name.vi"("Signal name"=refnum<k21> "Error_value\nCAN2_matrix_2022", "Signal list"=w541, "Signal data"=w540) -> ("Signal"=w573:dbl)
                  n242 = call "get_signal_by_name.vi"("Signal name"=refnum<k21> "HV_Acc_Menu\nCAN2_matrix_2022", "Signal list"=w541, "Signal data"=w540) -> ("Signal"=w578:dbl)
                  n243 = call "get_signal_by_name.vi"("Signal name"=refnum<k21> "HV_Cell_OT\nCAN2_matrix_2022", "Signal list"=w541, "Signal data"=w540) -> ("Signal"=w545:dbl)
                  n244 = call "get_signal_by_name.vi"("Signal name"=refnum<k21> "HV_Cell_OV\nCAN2_matrix_2022", "Signal list"=w541, "Signal data"=w540) -> ("Signal"=w544:dbl)
                  n245 = call "get_signal_by_name.vi"("Signal name"=refnum<k21> "HV_Cell_UV\nCAN2_matrix_2022", "Signal list"=w541, "Signal data"=w540) -> ("Signal"=w543:dbl)
                  n246 = call "get_signal_by_name.vi"("Signal name"=refnum<k21> "HV_DetStatus\nCAN2_matrix_2022", "Signal list"=w541, "Signal data"=w540) -> ("Signal"=w542:dbl)
                  n247 = call "get_signal_by_name.vi"("Signal name"=refnum<k21> "HV_ECU_Heartbeat\nCAN2_matrix_2022", "Signal list"=w541, "Signal data"=w540) -> ("Signal"=w539:dbl)
                  n248 = call "get_signal_by_name.vi"("Signal name"=refnum<k21> "HV_ECU_SC_Endline_State\nCAN2_matrix_2022", "Signal list"=w541, "Signal data"=w540) -> ("Signal"=w538:dbl)
                  n249 = call "get_signal_by_name.vi"("Signal name"=refnum<k21> "IMD_Relay_State\nCAN2_matrix_2022", "Signal list"=w541, "Signal data"=w540) -> ("Signal"=w537:dbl)
                  n250 = call "get_signal_by_name.vi"("Signal name"=refnum<k21> "IMD_Status\nCAN2_matrix_2022", "Signal list"=w541, "Signal data"=w540) -> ("Signal"=w536:dbl)
                  n251 = call "get_signal_by_name.vi"("Signal name"=refnum<k21> "MCU_STAMP\nCAN2_matrix_2022", "Signal list"=w541, "Signal data"=w540) -> ("Signal"=w535:dbl)
                  n252 = call "get_signal_by_name.vi"("Signal name"=refnum<k21> "PC_Error\nCAN2_matrix_2022", "Signal list"=w541, "Signal data"=w540) -> ("Signal"=w534:dbl)
                  n253 = call "get_signal_by_name.vi"("Signal name"=refnum<k21> "PC_State\nCAN2_matrix_2022", "Signal list"=w541, "Signal data"=w540) -> ("Signal"=w533:dbl)
                  n254 = call "get_signal_by_name.vi"("Signal name"=refnum<k21> "Place_of_error\nCAN2_matrix_2022", "Signal list"=w541, "Signal data"=w540) -> ("Signal"=w532:dbl)
                  n255 = call "get_signal_by_name.vi"("Signal name"=refnum<k21> "TSAL_GREEN\nCAN2_matrix_2022", "Signal list"=w541, "Signal data"=w540) -> ("Signal"=w531:dbl)
                  n256 = call "get_signal_by_name.vi"("Signal name"=refnum<k21> "TSAL_RED\nCAN2_matrix_2022", "Signal list"=w541, "Signal data"=w540) -> ("Signal"=w530:dbl)
                  n257 = call "get_signal_by_name.vi"("Signal name"=refnum<k21> "TS_Over_Voltage\nCAN2_matrix_2022", "Signal list"=w541, "Signal data"=w540) -> ("Signal"=w529:dbl)
                  n258 = call "get_signal_by_name.vi"("Signal name"=refnum<k21> "TS_Overcurrent\nCAN2_matrix_2022", "Signal list"=w541, "Signal data"=w540) -> ("Signal"=w528:dbl)
                  n259 = Bundle(cluster=T4 {"AIR_minus_state"=0.0, "AIR_plus_State"=0.0, "AMS_Relay_State"=0.0, "AMS_Status"=0.0, "Driver_Protection_State"=0.0, "Error_STAMP_TSAL"=0.0, "Error_value"=0.0, "HV_Acc_Menu"=0.0, "HV_Cell_OT"=0.0, "HV_Cell_OV"=0.0, "HV_Cell_UV"=0.0, "HV_DetStatus"=0.0, "HV_ECU_Heartbeat"=0.0, "HV_ECU_SC_Endline_State"=0.0, "IMD_Relay_State"=0.0, "IMD_Status"=0.0, "MCU_STAMP"=0.0, "PC_Error"=0.0, "PC_State"=0.0, "Place_of_error"=0.0, "TSAL_GREEN"=0.0, "TSAL_RED"=0.0, "TS_Over_Voltage"=0.0, "TS_Overcurrent"=0.0}, "AIR_minus_state"=w571, "AIR_plus_State"=w572, "AMS_Relay_State"=w577, "AMS_Status"=w576, "Driver_Protection_State"=w575, "Error_STAMP_TSAL"=w574, "Error_value"=w573, "HV_Acc_Menu"=w578, "HV_Cell_OT"=w545, "HV_Cell_OV"=w544, "HV_Cell_UV"=w543, "HV_DetStatus"=w542, "HV_ECU_Heartbeat"=w539, "HV_ECU_SC_Endline_State"=w538, "IMD_Relay_State"=w537, "IMD_Status"=w536, "MCU_STAMP"=w535, "PC_Error"=w534, "PC_State"=w533, "Place_of_error"=w532, "TSAL_GREEN"=w531, "TSAL_RED"=w530, "TS_Over_Voltage"=w529, "TS_Overcurrent"=w528) -> (→"530":T4)
                }
                frame 532 {
                  n260 = call "get_signal_by_name.vi"("Signal name"=refnum<k21> "HV_Voltage_Before_AIRs\nCAN2_matrix_2022", "Signal list"=w580, "Signal data"=w581) -> ("Signal"=w587:dbl)
                  n261 = call "get_signal_by_name.vi"("Signal name"=refnum<k21> "State_of_Charge\nCAN2_matrix_2022", "Signal list"=w580, "Signal data"=w581) -> ("Signal"=w588:dbl)
                  n262 = call "get_signal_by_name.vi"("Signal name"=refnum<k21> "HV_Current\nCAN2_matrix_2022", "Signal list"=w580, "Signal data"=w581) -> ("Signal"=w589:dbl)
                  n263 = call "get_signal_by_name.vi"("Signal name"=refnum<k21> "HV_Voltage_After_AIRs\nCAN2_matrix_2022", "Signal list"=w580, "Signal data"=w581) -> ("Signal"=w586:dbl)
                  n264 = Bundle(cluster=T3 {"HV_Current"=0.0, "HV_Voltage_After_AIRs"=0.0, "HV_Voltage_Before_AIRs"=0.0, "State_of_Charge"=0.0}, "HV_Current"=w589, "HV_Voltage_After_AIRs"=w586, "HV_Voltage_Before_AIRs"=w587, "State_of_Charge"=w588) -> (→"532":T3)
                }
                frame 528 {
                  n265 = call "get_signal_by_name.vi"("Signal name"=refnum<k21> "HV_Cell_Voltage\nCAN2_matrix_2022", "Signal list"=w591, "Signal data"=w592) -> ("Signal"=w597:dbl)
                  n266 = call "get_signal_by_name.vi"("Signal name"=refnum<k21> "HV_Cell_ID\nCAN2_matrix_2022", "Signal list"=w591, "Signal data"=w592) -> ("Signal"=w598:dbl)
                  n267 = call "get_signal_by_name.vi"("Signal name"=refnum<k21> "HV_Cell_Temperature\nCAN2_matrix_2022", "Signal list"=w591, "Signal data"=w592) -> ("Signal"=w596:dbl)
                  n268 = Bundle(cluster=T30 {"HV_Current"=0.0, "HV_Voltage_After_AIRs"=0.0, "HV_Voltage_Before_AIRs"=0.0}, "HV_Current"=w598, "HV_Voltage_After_AIRs"=w596, "HV_Voltage_Before_AIRs"=w597) -> ()  [unwired: 1 out]
                }
                frame 787 {
                  n269 = call "get_signal_by_name.vi"("Signal name"=refnum<k21> "HV_Cell_Voltage_MIN\nCAN2_matrix_2022", "Signal list"=w600, "Signal data"=w601) -> ("Signal"=w606:dbl)
                  n270 = call "get_signal_by_name.vi"("Signal name"=refnum<k21> "Critical_cell_values_heartbeat\nCAN2_matrix_2022", "Signal list"=w600, "Signal data"=w601) -> ("Signal"=w607:dbl)
                  n271 = call "get_signal_by_name.vi"("Signal name"=refnum<k21> "HV_Cell_Temp_MAX\nCAN2_matrix_2022", "Signal list"=w600, "Signal data"=w601) -> ("Signal"=w605:dbl)
                  n272 = Bundle(cluster=T30 {"HV_Current"=0.0, "HV_Voltage_After_AIRs"=0.0, "HV_Voltage_Before_AIRs"=0.0}, "HV_Current"=w607, "HV_Voltage_After_AIRs"=w605, "HV_Voltage_Before_AIRs"=w606) -> ()  [unwired: 1 out]
                }
                frame 393 {
                  n273 = call "get_signal_by_name.vi"("Signal name"=refnum<k21> "AMK3_TorqueLimitNegative\nCAN2_matrix_2022", "Signal list"=w610, "Signal data"=w611) -> ("Signal"=w617:dbl)
                  n274 = call "get_signal_by_name.vi"("Signal name"=refnum<k21> "AMK3_TorqueLimitPositive\nCAN2_matrix_2022", "Signal list"=w610, "Signal data"=w611) -> ("Signal"=w618:dbl)
                  n275 = call "get_signal_by_name.vi"("Signal name"=refnum<k21> "AMK3_Control\nCAN2_matrix_2022", "Signal list"=w610, "Signal data"=w611) -> ("Signal"=w619:dbl)
                  n276 = call "get_signal_by_name.vi"("Signal name"=refnum<k21> "AMK3_Target_Velocity\nCAN2_matrix_2022", "Signal list"=w610, "Signal data"=w611) -> ("Signal"=w616:dbl)
                  n277 = Bundle(cluster=T2 {"AMK3_Control"=0.0, "AMK3_Target_Velocity"=0.0, "AMK3_TorqueLimitNegative"=0.0, "AMK3_TorqueLimitPositive"=0.0}, "AMK3_Control"=w619, "AMK3_Target_Velocity"=w616, "AMK3_TorqueLimitNegative"=w617, "AMK3_TorqueLimitPositive"=w618) -> (→"393":T2)
                }
                frame 394 {
                  n278 = call "get_signal_by_name.vi"("Signal name"=refnum<k21> "AMK4_TorqueLimitNegative\nCAN2_matrix_2022", "Signal list"=w622, "Signal data"=w623) -> ("Signal"=w629:dbl)
                  n279 = call "get_signal_by_name.vi"("Signal name"=refnum<k21> "AMK4_TorqueLimitPositive\nCAN2_matrix_2022", "Signal list"=w622, "Signal data"=w623) -> ("Signal"=w630:dbl)
                  n280 = call "get_signal_by_name.vi"("Signal name"=refnum<k21> "AMK4_Control\nCAN2_matrix_2022", "Signal list"=w622, "Signal data"=w623) -> ("Signal"=w631:dbl)
                  n281 = call "get_signal_by_name.vi"("Signal name"=refnum<k21> "AMK4_Target_Velocity\nCAN2_matrix_2022", "Signal list"=w622, "Signal data"=w623) -> ("Signal"=w628:dbl)
                  n282 = Bundle(cluster=T1 {"AMK4_Control"=0.0, "AMK4_Target_Velocity"=0.0, "AMK4_TorqueLimitNegative"=0.0, "AMK4_TorqueLimitPositive"=0.0}, "AMK4_Control"=w631, "AMK4_Target_Velocity"=w628, "AMK4_TorqueLimitNegative"=w629, "AMK4_TorqueLimitPositive"=w630) -> (→"394":T1)
                }
                frame 401 {
                  n283 = call "get_signal_by_name.vi"("Signal name"=refnum<k21> "RES_GO_Signal\nCAN2_matrix_2022", "Signal list"=w635, "Signal data"=w636) -> ("Signal"=→"401":dbl)
                }
              }
            }
          }
        }
      }
      frame #2 {
        n284 = Tick Count (ms)() -> (millisecond timer value=w689:u32)
        n285 = Subtract(x=w689, y=w690) -> (x-y=→"Actual Timestep":u32)
      }
    }
    "Is running" <- "?"
  }
  n286 = String To IP(1:"ip") -> (0:w2:u32)
  n287 = UDP Open(11:u16 0 ("port")) -> (port=w5:refnum<k16>)  [unwired: 4 in, 2 out]
  n288 = while {
    tunnel: w14 -> [w697]
    tunnel: w16 -> [w696]
    tunnel: "Main timestep" -> [w694]
    tunnel: w5 -> [w693]
    tunnel: "Port" -> [w692]
    tunnel: w2 -> [w691]
    i -> [w699]
    stop <- FALSE stop-if-true
    n289 = Wait Until Next ms Multiple(millisecond multiple=w694) -> ()  [unwired: 1 out]
    n290 = case shown="True" "stresstest" {
      tunnel: w699 -> [_ w712]
      tunnel: w697 -> [_ w709]
      tunnel: w696 -> [_ w708]
      tunnel: w693 -> [_ w704]
      tunnel: w692 -> [_ w702]
      tunnel: w691 -> [_ w700]
      frame False {
      }
      frame True {
        n291 = Quotient & Remainder(x=w712, y=2) -> (x-y*floor(x/y)=w710:i32)  [unwired: 1 out]
        n292 = flat-sequence {
          tunnel: [w722] -> w715
          tunnel: w710 -> [w722]
          tunnel: [w720] -> w714
          tunnel: [w721] -> w713
          tunnel: w709 -> [w721]
          tunnel: w708 -> [w720]
          tunnel: [w719] -> w706
          tunnel: [w718] -> w705
          tunnel: w704 -> [w718]
          tunnel: [w717] -> w703
          tunnel: w702 -> [w717]
          tunnel: [w716] -> w701
          tunnel: w700 -> [w716]
          tunnel: w715 -> [w731]
          tunnel: w714 -> [w730]
          tunnel: w713 -> [w729]
          tunnel: [w727] -> w707
          tunnel: w706 -> [w727]
          tunnel: w705 -> [w725]
          tunnel: w703 -> [w724]
          tunnel: w701 -> [w723]
          tunnel: w707 -> [w735]
          frame #0 {
            n293 = Tick Count (ms)() -> (millisecond timer value=w719:u32)
          }
          frame #1 {
            n294 = case shown="0, Default" w731 {
              tunnel: [w732 w733] -> w728
              tunnel: w730 -> [w732 _]
              tunnel: w729 -> [_ w733]
              frame 0, Default {
              }
              frame 1 {
              }
            }
            n295 = Byte Array To String(unsigned byte array=w728) -> (string=w726:string)
            n296 = UDP Write(address=w723, port or service name=w724, connection ID=w725, data in=w726) -> ()  [unwired: 2 in, 2 out]
          }
          frame #2 {
            n297 = Tick Count (ms)() -> (millisecond timer value=w736:u32)
            n298 = Subtract(x=w736, y=w735) -> (x-y=→"UDP timestep":u32)
          }
        }
      }
    }
  }
